vi "DB Manager.vi"(8 "error in":errorcluster caption="에러 입력(에러 없음)") -> (0 "error out":errorcluster caption="에러 출력")   [LabVIEW 2020]
uses:
  Support/Controls/Cmd_Mouse Popup.ctl
  Support/Controls/Clst_DBM data.ctl
  Support/Controls/Clst_Query Info.ctl
  <vilib>/Utility/miscctls.llb/LVRowAndColumnUnsignedTypeDef.ctl
  <vilib>/Utility/NIReport.llb/Report Type.ctl
  Support/Controls/Cmd_Read Query.ctl
  Support/Controls/Cmd_Write Query.ctl
  Variables/Global_Cal Info.vi
  Support/Public/Polymorph/Cell Space_ListBox.vi
  Support/Public/Polymorph/Data Class_2D Str.vi
  Support/Public/Polymorph/Cell Space_Table.vi
  <vilib>/Utility/error.llb/Error Cluster From Error Code.vi
  <vilib>/addons/_office/excel.llb/Excel Get Data (str).vi
  Support/Public/Polymorph/Array Dedup_1D Str.vi
  <vilib>/ErrorRing/Error Ring.xnode
  <vilib>/addons/database/NI_Database_API.lvlib
  <vilib>/Utility/NIReport.llb/NI_report.lvclass
  <vilib>/Utility/NIReport.llb/NI_ReportGenerationCore.lvlib
  <vilib>/addons/_office/NI_ReportGenerationToolkit.lvlib
  <vilib>/Utility/NIReport.llb/Excel/NI_Excel.lvclass
panel:
  out "Data":string[][](array[string])
  out "모델등록요청":u8
  out "기준기등록요청":u8
  in  "TOP_요청삭제":bool
  in  "TOP_등록요청":bool
  in  "TOP_추가":bool
  in  "TOP_항목명":u16(ring) caption="항목명" items=["ALL [ - ]", "10201-0 [ 볼; 강구, 표준구 등 ]", "10203-0 [ 기계/전기식 콤퍼레이터 ]", "10206-0 [ 다이얼/실린더 게이지 시험기 ]", "10207-0 [ 닥터 블레이드 ]", "10209-0 [ 엔드바, 마이크로미터 기준봉 ]", "10210-1 [ 길이 변위계 ]", "10210-2 [ LVDT ]", "10211-0 [ 틈새 게이지 ]", "10212-0 [ 필름 어플리케이터 ]", "10213-0 [ 갭 게이지 ]", "10214-0 [ 게이지 블록, 비교교정 ]", "10216-0 [ 높이 게이지/측정기 ]", "10219-0 [ 리니어 스케일 ]", "10220-0 [ 표준 측장기 ]", "10223-0 [ 전기 마이크로미터 ]", "10224-1 [ 높이 마이크로미터 ]", "10224-2 [ 받침블록 ]", "10225-0 [ 레이저 스캔 마이크로미터 ]", "10227-0 [ 표준 내/외경 줄자 ]", "10228-1 [ 원통형 플러그 게이지 ]", "10228-2 [ 핀 게이지 ]", "10229-0 [ 래디어스 게이지 ]", "10230-0 [ 원통형 링 게이지 ]", "10231-0 [ 게이지 블록 단차시편 ]", "10232-1 [ 스텝 게이지 ]", "10232-2 [ 캘리퍼 검사기 ]", "10233-0 [ 테이퍼형 틈새 게이지 ]", "10234-0 [ 초음파식 두께 측정기 ]", "10235-1 [ 두께 측정용 기준시편; 코팅형 ]", "10235-2 [ 두께 측정용 기준시편; 초음파 시편 ]", "10236-0 [ 피막 두께 측정기 ]", "10237-0 [ 토크 암 ]", "10238-0 [ 폭 측정용 기준 시편 ]", "10304-1 [ 각도정규 ]", "10304-2 [ 디지털 각도기 ]", "10311-1 [ 전기식 수준기 ]", "10311-2 [ 평형/각형 수준기 ]", "10317-0 [ 사인바, 플레이트, 테이블, 센터 ]", "10318-0 [ 직각도 시험기 ]", "10319-0 [ 원통 스퀘어 ]", "10320-0 [ 정밀직각기준, 직각자 ]", "10401-0 [ 형상 측정기 ]", "10404-0 [ 옵티컬 플랫 ]", "10405-0 [ 옵티컬 파라렐 ]", "10406-0 [ 평행블록 ]", "10407-0 [ 정밀 정반 ]", "10409-0 [ 진원도 측정기 ]", "10412-0 [ 스트레이트 엣지 ]", "10413-0 [ 곧은자 ]", "10415-0 [ 테스트 바아 ]", "10416-0 [ 구면계 ]", "10503-0 [ 접촉식 좌표 측정기 ]", "10504-1 [ 비접촉식 좌표 측정기 ]", "10504-2 [ 화상측정기 ]", "10505-0 [ 게이지 블록 부속품 ]", "10511-1 [ 측정현미경 ]", "10511-2 [ 측정투영기 ]", "10511-3 [ 측정 현미경 (영상) ]", "10512-0 [ 측미 현미경 ]", "10517-0 [ 촉침식 표면 거칠기 측정기 ]", "10525-0 [ 나사 플러그 게이지 ]", "10529-0 [ 브이블록 및 박스블록 ]", "10601-1 [ 내/외측 캘리퍼 ]", "10601-3 [ 캘리퍼 게이지 ]", "10603-1 [ 실린더 게이지 ]", "10603-2 [ 보어 게이지 ]", "10604-1 [ 깊이 게이지 ]", "10604-2 [ 깊이마이크로미터 ]", "10605-1 [ 다이얼/디지털 게이지 ]", "10605-2 [ 다이얼 및 디지털 두께 측정기 ]", "10609-1 [ 지침 측미기 ]", "10609-2 [ 테스트 인디케이터 ]", "10610-0 [ 마이크로미터 헤드 ]", "10611-0 [ 3점 마이크로미터 ]", "10612-1 [ 내측 마이크로미터 ]", "10612-2 [ 봉형 내측 마이크로미터 ]", "10613-1 [ 외측 마이크로미터 ]", "10613-2 [ V-앤빌 마이크로미터 ]", "10613-3 [ 벤치 마이크로미터 ]", "10615-1 [ 공기입자계수기 ]", "10615-2 [ 액체 입자계수기 ]", "10617-0 [ 표준체 ]", "10620-0 [ 용접 게이지 ]", "10622-0 [ 입자희석장치 ]", "20105-0 [ 부등비 접시 수동 저울 ]", "20106-0 [ 판 지시 저울 ]", "20108-0 [ 반 지시 맞 저울 ]", "20109-0 [ 전기식 지시 저울 ]", "20112-0 [ 판수동/플랫트 폼 저울 ]", "20113-0 [ 접시 지시저울,스프링 지시 저울 ]", "20116-1 [ 분동 ]", "20116-2 [ 추 ]", "20202-0 [ 힘 측정기 ]", "20203-0 [ 인장 및 압축 시험기 ]", "20204-0 [ 푸쉬풀 게이지 ]", "20302-0 [ 토크 측정기 ]", "20303-0 [ 토크 렌치 및 토크 드라이버 ]", "20402-0 [ 액주형 압력계 ]", "20406-0 [ 절대압계 ]", "20408-0 [ 연성 압력계 ]", "20409-0 [ 차압계 ]", "20411-1 [ 게이지압용 압력계 ]", "20411-2 [ AUTOCLAVE, HAST CHAMBER(지시계포함) ]", "20411-3 [ 압력조절기 ]", "20411-4 [ 압력기록계 ]", "20412-1 [ 압력 변환기/전송기(게이지압) ]", "20412-2 [ 압력 변환기/전송기(절대압) ]", "20412-3 [ 압력 변환기/전송기(차압) ]", "20413-0 [ 다이얼형 진공계 ]", "20414-0 [ 수심계 ]", "20601-0 [ 유리제 부피계; 타 재질 포함 ]", "20602-0 [ 비중병; 스테인리스 스틸 포함 ]", "20605-0 [ 콘크리트 공기량 시험기 ]", "20606-0 [ 피스톤식 부피계 ]", "20802-0 [ 회전형 점도계 ]", "20901-1 [ 열선형 유속계 ]", "20901-2 [ 열선형 유속계(센서형) ]", "20902-0 [ 피토관 유속계 ]", "20908-0 [ 기체용 차압 유량계 ]", "20909-0 [ 액체용 차압 유량계 ]", "20910-0 [ 액체용 전자기 유량계 ]", "20911-0 [ 기체용 질량 유량계 ]", "20912-0 [ 액체용 질량 유량계 ]", "20914-0 [ 기체용 용적 유량계 ]", "20915-0 [ 액체용 용적 유량계 ]", "20916-0 [ 기체용 터빈 유량계 ]", "20917-0 [ 액체용 터빈 유량계 ]", "20918-0 [ 기체용 초음파 유량계 ]", "20919-0 [ 액체용 초음파 유량계 ]", "20920-0 [ 기체용 면적 유량계 ]", "20921-0 [ 액체용 면적 유량계 ]", "20922-0 [ 기체용 와 유량계 ]", "20923-0 [ 액체용 와 유량계 ]", "20925-0 [ 회전형 유속계 ]", "30102-1 [ 주파수 표준기 ]", "30102-2 [ 주파수 비교기 ]", "30103-0 [ 주파수 발생기 ]", "30104-1 [ 주파수 계수기 ]", "30104-2 [ 주파수 계수기 플러그 유니트 ]", "30104-3 [ 상용 주파수계 ]", "30104-4 [ 주파수 계 ]", "30105-1 [ 시간간격 발생기 ]", "30105-2 [ 주파수 발생기 ]", "30106-1 [ 시간간격 측정기 ]", "30106-2 [ 초시계 ]", "30106-3 [ 타이머 ]", "30106-4 [ 카운터 ]", "30201-0 [ 표준 회전속도 발생장치 ]", "30202-0 [ 접촉식 회전 속도계 ]", "30203-0 [ 광 회전 속도계 ]", "30205-0 [ 와우-후러터 발생장치 ]", "30206-0 [ 와우-후러터 미터 ]", "40101-0 [ 직류 전류계 ]", "40102-0 [ 직류 전압전류 변환기 ]", "40103-0 [ 직류 전압/전류 교정기 ]", "40104-0 [ 전기식 온도 교정기 ]", "40105-0 [ 직류용 분류기 ]", "40106-0 [ 검류계 ]", "40108-0 [ 직류 전원 공급기 ]", "40110-0 [ 직류 전압 분할기 ]", "40111-0 [ 전자형 직류 기준전압 ]", "40112-1 [ 직류 전압계 ]", "40112-2 [ 차동 전압계 등 ]", "40113-1 [ 정전기 측정기 ]", "40113-2 [ 이온 측정기 ]", "40201-1 [ 용량 브리지 ]", "40201-2 [ 용량 지시기 ]", "40202-0 [ 계단식 용량기 ]", "40204-0 [ 표준 용량기 ]", "40205-0 [ 접지 저항 측정기 ]", "40208-1 [ 유도기 ]", "40208-2 [ 계단식 유도기 ]", "40210-0 [ 절연시험기 ]", "40211-0 [ Q-미터 ]", "40213-1 [ 저항 브리지 ]", "40213-2 [ 저항 유사장비 ]", "40214-0 [ 저항 측정기 ]", "40215-1 [ 표준 저항기 ]", "40215-2 [ 계단식 저항기 ]", "40216-1 [ 전기전도도 미터 ]", "40216-2 [ 전도도 미터 ]", "40217-1 [ LCR 미터 ]", "40217-2 [ 임피던스 브리지 ]", "40301-0 [ 교류 전류계 ]", "40302-1 [ 클램프형  전류계/전압계 ]", "40302-2 [ 전류코일 ]", "40303-0 [ 교류 전압/전류 교정기 ]", "40304-0 [ 전력계 교정기 ]", "40305-0 [ 교류 전류 분류기 ]", "40310-1 [ 역률계 ]", "40310-2 [ 무효율계 ]", "40311-0 [ 교류 전력계 ]", "40312-0 [ 교류 전원 공급기 ]", "40313-0 [ 내전압/전기 안전 시험기 ]", "40314-0 [ 전력 기록계 ]", "40318-0 [ 교류 전압계/전위차, 실효치 ]", "40401-1 [ 저주파 증폭기 ]", "40401-2 [ 챠지/전압 증폭기 ]", "40402-0 [ 직류/저주파 감쇠기 ]", "40403-0 [ 멀티미터 교정기 ]", "40404-0 [ 파형 측정기 교정기 ]", "40406-0 [ 영상 신호 발생기 ]", "40407-1 [ 오디오 분석기 ]", "40407-2 [ 왜율 미터 ]", "40408-0 [ 저주파용 여파기 ]", "40409-0 [ 저주파 신호 분석기 ]", "40410-0 [ 전원 주파수계 ]", "40411-1 [ 다기능 파형 발생기 ]", "40411-2 [ 구형파 발생기 ]", "40412-0 [ 제네스코프 ]", "40413-0 [ 직·교류 고전압계 ]", "40416-0 [ 누설전류 시험기 ]", "40417-0 [ 직/교류 전자부하 ]", "40419-0 [ 멀티미터 ]", "40420-0 [ 잡음 전압 측정기 ]", "40421-0 [ 파형 측정기 ]", "40422-0 [ 저주파 위상계 ]", "40423-0 [ 랜덤파형 발생기 ]", "40424-0 [ 전압 전류 기록계 ]", "40425-0 [ 릴레이 시험기 ]", "40426-0 [ LF 신호 발생기 ]", "40427-0 [ 저주파 스펙트럼 분석기 ]", "40429-0 [ 스위프 발생기 ]", "40432-0 [ 트란지스터 특성 곡선 측정기 ]", "40433-0 [ 파형 분석기 ]", "40434-0 [ 직/교류 고전압 출력기 ]", "40435-0 [ 직/교류 고전압 프로브 ]", "40436-0 [ 논리 회로분석기 ]", "40437-0 [ 전화기 시험기 ]", "40438-0 [ 영상 신호 분석기 ]", "40503-0 [ 자속 미터 ]", "40504-0 [ 플럭스 원 ]", "40508-0 [ 마그네토 미터 ]", "40510-0 [ 표준 자석 ]", "40601-0 [ 고주파 증폭기 ]", "40602-1 [ 동축형 고정 감쇠기 ]", "40602-2 [ 동축형 가변 감쇠기 ]", "40603-1 [ 도파관형 고정 감쇠기 ]", "40603-2 [ 도파관형 가변 감쇠기 ]", "40605-0 [ 버스트 펄스 발생기 ]", "40606-0 [ 감쇠기 교정기 ]", "40607-0 [ 고주파 전력 측정기 교정기 ]", "40608-1 [ EMC용 변환기 ]", "40608-2 [ 흡수 클램프 ]", "40610-0 [ 동축형 방향성 결합기/분배기 ]", "40611-0 [ 도파관형 방향성 결합기 ]", "40613-0 [ 정전기 발생기 ]", "40614-0 [ EMC 수신기 ]", "40615-0 [ 고주파/전자파 여파기 ]", "40616-0 [ 고주파 임피던스 미터 ]", "40617-0 [ 고주파 스펙트럼 분석기 ]", "40618-1 [ 전원 임피던스 안정화 회로망 ]", "40618-2 [ 결합 감결합 회로망 ]", "40618-3 [ 임피던스 안정화 회로망 ]", "40618-4 [ 전자기 클램프 ]", "40618-5 [ 임피던스 변환기 ]", "40619-1 [ 동축형 표준 부정합 ]", "40621-0 [ 이동통신 종합시험기 ]", "40622-0 [ 변조계 ]", "40623-0 [ 회로망 분석기 ]", "40624-0 [ 잡음계수 측정기 ]", "40625-0 [ 잡음 발생기 ]", "40626-0 [ 잡음 충격파 시험기 ]", "40635-1 [ 고주파 전력 측정기 ]", "40635-2 [ 고주파 고전력계 ]", "40636-0 [ 다이오드 전력 감지기 ]", "40637-0 [ 열전대 전력 감지기 ]", "40638-0 [ 펄스 발생기 ]", "40639-1 [ 레이더 시험장치 ]", "40639-2 [ 레이더 시험장치 ]", "40639-3 [ 레이더 시험장치 ]", "40639-4 [ 레이더 시험장치 ]", "40639-5 [ 레이더 시험장치 ]", "40640-0 [ 고주파 신호 발생기 ]", "40641-1 [ 고주파 스펙트럼 분석기 ]", "40641-2 [ FFT 분석기 ]", "40642-0 [ 속도 측정기 ]", "40643-0 [ 서지 발생기 ]", "40645-0 [ 고주파 터미네이션 ]", "40646-0 [ 동축형 서미스터 마운트 ]", "40648-0 [ 전송 장애 측정 시험기 ]", "40650-0 [ 고주파 전압계 ]", "40651-0 [ 벡터 전압계 ]", "40652-0 [ 전자기장의 세기 측정기 ]", "40653-0 [ 측정 수신기 ]", "40654-0 [ 딥 시뮬레이터 ]", "40701-0 [ 누설 전자파 측정기 ]", "40702-1 [ 프로브 류-전계 프로브 ]", "40702-2 [ 프로브 류-자계 프로브 ]", "40703-1 [ 이극 안테나 류-SAR 측정용 전기장 프로브 ]", "40703-2 [ 이극 안테나 류-SAR 측정용 다이폴 안테나 ]", "40703-3 [ 이극 안테나 류-다이폴 안테나 ]", "40703-4 [ 이극 안테나 류-바이코니컬 안테나 ]", "40703-5 [ 이극 안테나 류-대수주기 안테나 ]", "40703-6 [ 이극 안테나 류-하이브리드 안테나 ]", "40704-0 [ 환상 안테나 류 ]", "40705-0 [ 단극 안테나 류 ]", "40707-0 [ 혼 안테나 류 ]", "50101-1 [ 온도 조절형 챔버 및 오븐 ]", "50101-2 [ 전기로 ]", "50101-3 [ 액체항온조 ]", "50101-4 [ 빙점조 ]", "50101-5 [ 드라이블럭교정기 ]", "50102-1 [ 온도 지시계(센서포함_열전식) ]", "50102-2 [ 온도 지시계(센서미포함_열전식) ]", "50102-3 [ 온도 지시계(센서미포함_저항식) ]", "50102-4 [ 온도 지시계(센서포함_저항식) ]", "50103-0 [ 유리제 온도계 ]", "50104-0 [ 저항식 온도계 ]", "50105-0 [ 열팽창식 온도계 ]", "50106-1 [ 열전대(귀금속) ]", "50106-2 [ 열전대(비금속) ]", "50107-0 [ 온도 변환기 ]", "50204-0 [ 복사온도계 ]", "50205-0 [ 복사열 영상측정장치 ]", "50206-0 [ 흑체로 ]", "50301-0 [ 알루미나 박막습도계 ]", "50302-1 [ 고분자 박막습도계 ]", "50302-2 [ 모발 습도계 ]", "50302-3 [ 디지털온습도계 ]", "50304-0 [ 온도/습도 기록계 ]", "50305-0 [ 상대습도 변환기 ]", "50306-1 [ 분류식 습도발생장치 ]", "50306-2 [ 항온항습기 ]", "60102-1 [ 다기능 음향 교정기 ]", "60102-2 [ 피스톤폰 ]", "60102-3 [ 음압 레벨교정기 ]", "60104-1 [ 마이크로폰 ]", "60104-2 [ 마이크로폰(3단자 결합기) ]", "60106-1 [ 소음계 ]", "60106-2 [ 소음계 ]", "60301-0 [ 진동계 교정기 ]", "60302-1 [ 진동 변환기 ]", "60302-2 [ 충격 변환기 ]", "60303-1 [ 진동 측정기 ]", "60303-2 [ 충격 측정기 ]", "70101-0 [ 광조도계 ]", "70102-0 [ 광휘도계 ]", "70103-0 [ 전광선속계 ]", "70104-0 [ 광도계 ]", "70202-0 [ 색온도측정기 ]", "70203-0 [ 색온도 표준전구 ]", "70204-0 [ 색채계; 광원색 ]", "70209-0 [ 전광선속 표준전구 ]", "70213-0 [ 디스플레이 색채 분석기; 광휘도, 색좌표, 화이트밸런스 등 ]", "70214-0 [ 광도 표준전구 ]", "70215-0 [ 분광복사조도 표준전구 ]", "70216-0 [ 전분광복사선속 표준전구 ]", "70217-0 [ 광휘도 표준광원 ]", "70218-0 [ 분광복사휘도 표준광원 ]", "70219-0 [ 자외선 복사조도계 ]", "70220-0 [ 분광복사조도계 ]", "70221-0 [ 전분광복사선속계 ]", "70222-0 [ 분광복사휘도계 ]", "70223-0 [ 분광복사도계 ]", "70402-0 [ 광대역광원 ]", "70410-0 [ 광감쇠기 ]", "70413-0 [ 광감쇠량측정기 ]", "70415-0 [ 광 멀티미터 ]", "70417-0 [ 광스펙트럼 분석기 ]", "70418-0 [ 시간영역 광반사계 ]", "70430-0 [ ASE 광원 ]", "70433-0 [ 광출력 안정화 레이저 및 LDs ]", "90102-0 [ 대기가스 감시기 ]", "90103-0 [ 가스 분석기 ]", "90104-0 [ 배기가스 측정기 ]", "N0001-0 [ INSPECTION JIG & FIXTURE ]", "N0002-0 [ 진동시험기 ]"]
  in  "TOP_삭제":bool
  in  "TOP_파일생성":bool
  in  "TOP_등록":bool
  in  "TOP_조회":bool
  in  "TOP_초기화":bool
  in  "TOP_종료":bool
  out "Func":string
  out "SubVI List":string[](array[string])
  out "슬라이드":u32(slide) scale=-1.0..3.0
  out "교정기능목록":string[][](array[string])
  out "세부분류목록":string[][](array[string])=[["ALL", "-"], ["10201-0", "볼; 강구, 표준구 등"], ["10206-0", "다이얼/실린더 게이지 시험기"], ["10209-0", "엔드바, 마이크로미터 기준봉"], ["10210-1", "길이 변위계"], ["10210-2", "LVDT"], ["10210-3", "길이 변위계"], ["10211-0", "틈새 게이지"], ["10213-0", "갭 게이지"], ["10214-0", "게이지 블록, 비교교정"], ["10216-0", "높이 게이지/측정기"], ["10220-0", "표준 측장기"], ["10223-0", "전기 마이크로미터"], ["10224-1", "높이 마이크로미터"], ["10224-2", "받침블록"], ["10227-0", "표준 내/외경 줄자"], ["10228-1", "원통형 플러그 게이지"], ["10228-2", "핀 게이지"], ["10229-0", "래디어스 게이지"], ["10230-0", "원통형 링 게이지"], ["10232-1", "스텝 게이지"], ["10232-2", "캘리퍼 검사기"], ["10233-0", "테이퍼형 틈새 게이지"], ["10234-0", "초음파식 두께 측정기"], ["10235-0", "두께 측정용 기준시편;코팅형, 초음파 시편"], ["10236-0", "피막 두께 측정기"], ["10304-1", "각도정규"], ["10304-2", "콤비네이션셋"], ["10311-1", "전기식 수준기"], ["10311-2", "평형/각형 수준기"], ["10404-0", "옵티컬 플랫"], ["10405-0", "옵티컬 파라렐"], ["10407-0", "정밀 정반"], ["10413-0", "곧은자"], ["10503-0", "접촉식 좌표 측정기"], ["10504-0", "비접촉식 좌표 측정기"], ["10511-1", "측정현미경"], ["10511-2", "측정투영기"], ["10511-3", "측정 현미경 (영상)"], ["10512-0", "측미 현미경"], ["10525-0", "나사 플러그 게이지"], ["10601-1", "내/외측 캘리퍼"], ["10601-3", "캘리퍼 게이지"], ["10603-1", "실린더 게이지"], ["10603-2", "보어 게이지"], ["10604-1", "깊이 게이지"], ["10604-2", "깊이마이크로미터"], ["10605-0", "다이얼/디지털 게이지"], ["10609-1", "지침 측미기"], ["10609-2", "테스트 인디케이터"], ["10610-0", "마이크로미터 헤드"], ["10611-0", "3점 마이크로미터"], ["10612-1", "내측 마이크로미터"], ["10612-2", "봉형 내측 마이크로미터"], ["10613-1", "외측 마이크로미터"], ["10615-1", "공기입자계수기"], ["10615-2", "액체 입자계수기"], ["10617-0", "표준체"], ["10620-0", "용접 게이지"], ["10622-0", "입자희석장치"], ["20105-0", "부등비 접시 수동 저울"], ["20108-0", "반 지시 맞 저울"], ["20109-0", "전기식 지시 저울"], ["20112-0", "판수동/플랫트 폼 저울"], ["20113-0", "접시 지시저울,스프링 지시 저울"], ["20116-1", "분동"], ["20116-2", "추"], ["20202-0", "힘 측정기"], ["20203-0", "인장 및 압축 시험기"], ["20204-0", "푸쉬풀 게이지"], ["20302-0", "토크 측정기"], ["20303-0", "토크 렌치 및 토크 드라이버"], ["20406-0", "절대압계"], ["20408-0", "연성 압력계"], ["20409-0", "차압계"], ["20411-1", "게이지압용 압력계"], ["20411-2", "압력 발생기"], ["20411-3", "압력 조절기"], ["20411-4", "압력기록계"], ["20412-0", "압력 변환기/전송기"], ["20413-0", "다이얼형 진공계"], ["20414-0", "수심계"], ["20901-1", "열선형 유속계"], ["20901-2", "열선형 유속계(센서형)"], ["20902-0", "피토관 유속계"], ["20925-0", "회전형 유속계"], ["30102-1", "주파수 표준기"], ["30102-2", "주파수 비교기"], ["30103-0", "주파수 발생기"], ["30104-1", "주파수 계수기"], ["30104-2", "주파수 계수기 플러그 유니트"], ["30104-3", "상용 주파수계"], ["30104-4", "주파수 계"], ["30105-1", "시간간격 발생기"], ["30105-2", "주파수 발생기"], ["30106-1", "시간간격 측정기"], ["30106-2", "초시계"], ["30106-3", "타이머"], ["30201-0", "표준 회전속도 발생장치"], ["30202-0", "접촉식 회전 속도계"], ["30203-0", "광 회전 속도계"], ["30205-0", "와우-후러터 발생장치"], ["30206-0", "와우-후러터 미터"], ["40101-0", "직류 전류계"], ["40102-0", "직류 전압전류 변환기"], ["40103-0", "직류 전압/전류 교정기"], ["40104-0", "전기식 온도 교정기"], ["40105-0", "직류용 분류기"], ["40106-0", "검류계"], ["40108-0", "직류 전원 공급기"], ["40111-0", "전자형 직류 기준전압"], ["40112-1", "직류 전압계"], ["40112-2", "차동 전압계 등"], ["40113-1", "정전기 측정기"], ["40113-2", "이온 측정기"], ["40201-1", "용량 브리지"], ["40201-2", "용량 지시기"], ["40202-0", "계단식 용량기"], ["40204-0", "표준 용량기"], ["40205-0", "접지 저항 측정기"], ["40208-1", "유도기"], ["40208-2", "계단식 유도기"], ["40210-0", "절연시험기"], ["40211-0", "Q-미터"], ["40213-1", "저항 브리지"], ["40213-2", "저항 유사장비"], ["40214-0", "저항 측정기"], ["40215-1", "표준 저항기"], ["40215-2", "계단식 저항기"], ["40216-1", "전기전도도 미터"], ["40216-2", "전도도 미터"], ["40217-1", "LCR 미터"], ["40217-2", "임피던스 브리지"], ["40301-0", "교류 전류계"], ["40302-1", "클램프형  전류계/전압계"], ["40302-2", "전류코일"], ["40303-0", "교류 전압/전류 교정기"], ["40305-0", "교류 전류 분류기"], ["40310-1", "역률계"], ["40310-2", "무효율계"], ["40311-0", "교류 전력계"], ["40312-0", "교류 전원 공급기"], ["40313-0", "내전압/전기 안전 시험기"], ["40314-0", "전력 기록계"], ["40318-0", "교류 전압계/전위차, 실효치"], ["40401-1", "저주파 증폭기"], ["40401-2", "챠지/전압 증폭기"], ["40402-0", "직류/저주파 감쇠기"], ["40403-0", "멀티미터 교정기"], ["40404-0", "파형 측정기 교정기"], ["40406-0", "영상 신호 발생기"], ["40407-1", "오디오 분석기"], ["40407-2", "왜율 미터"], ["40408-0", "저주파용 여파기"], ["40409-0", "저주파 신호 분석기"], ["40410-0", "전원 주파수계"], ["40411-1", "다기능 파형 발생기"], ["40411-2", "구형파 발생기"], ["40412-0", "제네스코프"], ["40413-0", "직·교류 고전압계"], ["40416-0", "누설전류 시험기"], ["40417-0", "직/교류 전자부하"], ["40419-0", "멀티미터"], ["40420-0", "잡음 전압 측정기"], ["40421-0", "파형 측정기"], ["40422-0", "저주파 위상계"], ["40423-0", "랜덤파형 발생기"], ["40424-0", "전압 전류 기록계"], ["40425-0", "릴레이 시험기"], ["40426-0", "LF 신호 발생기"], ["40427-0", "저주파 스펙트럼 분석기"], ["40429-0", "스위프 발생기"], ["40432-0", "트란지스터 특성 곡선 측정기"], ["40433-0", "파형 분석기"], ["40434-0", "직/교류 고전압 출력기"], ["40435-0", "직/교류 고전압 프로브"], ["40436-0", "논리 회로분석기"], ["40437-0", "전화기 시험기"], ["40438-0", "영상 신호 분석기"], ["40503-0", "자속 미터"], ["40504-0", "플럭스 원"], ["40508-0", "마그네토 미터"], ["40510-0", "표준 자석"], ["40601-0", "고주파 증폭기"], ["40602-1", "동축형 고정 감쇠기"], ["40602-2", "동축형 가변 감쇠기"], ["40605-0", "버스트 펄스 발생기"], ["40606-0", "감쇠기 교정기"], ["40607-0", "고주파 전력 측정기 교정기"], ["40608-1", "EMC용 변환기"], ["40608-2", "흡수 클램프"], ["40610-0", "동축형 방향성 결합기/분배기"], ["40613-0", "정전기 발생기"], ["40614-0", "EMC 수신기"], ["40615-0", "고주파/전자파 여파기"], ["40616-0", "고주파 임피던스 미터"], ["40617-0", "고주파 스펙트럼 분석기"], ["40618-1", "전원 임피던스 안정화 회로망"], ["40618-2", "결합 감결합 회로망"], ["40618-3", "임피던스 안정화 회로망"], ["40618-4", "전자기 클램프"], ["40618-5", "임피던스 변환기"], ["40619-1", "동축형 표준 부정합"], ["40621-0", "이동통신 종합시험기"], ["40622-0", "변조계"], ["40623-0", "회로망 분석기"], ["40624-0", "잡음계수 측정기"], ["40625-0", "잡음 발생기"], ["40626-0", "잡음 충격파 시험기"], ["40635-1", "고주파 전력 측정기"], ["40635-2", "고주파 고전력계"], ["40636-0", "다이오드 전력 감지기"], ["40637-0", "열전대 전력 감지기"], ["40638-0", "펄스 발생기"], ["40639-0", "레이더 시험장치"], ["40640-0", "고주파 신호 발생기"], ["40641-1", "고주파 스펙트럼 분석기"], ["40641-2", "FFT 분석기"], ["40642-0", "속도 측정기"], ["40643-0", "서지 발생기"], ["40645-0", "고주파 터미네이션"], ["40646-0", "동축형 서미스터 마운트"], ["40648-0", "전송 장애 측정 시험기"], ["40650-0", "고주파 전압계"], ["40651-0", "벡터 전압계"], ["40652-0", "전자기장의 세기 측정기"], ["40653-0", "측정 수신기"], ["40654-0", "딥 시뮬레이터"], ["40702-1", "프로브 류-전계 프로브"], ["40702-2", "프로브 류-자계 프로브"], ["40703-1", "이극 안테나 류-SAR 측정용 전기장 프로브"], ["40703-2", "이극 안테나 류-SAR 측정용 다이폴 안테나"], ["40703-3", "이극 안테나 류-다이폴 안테나"], ["40703-4", "이극 안테나 류-바이코니컬 안테나"], ["40703-5", "이극 안테나 류-대수주기 안테나"], ["40703-6", "이극 안테나 류-하이브리드 안테나"], ["40704-0", "환상 안테나 류"], ["40705-0", "단극 안테나 류"], ["40707-0", "혼 안테나 류"], ["50101-1", "온도 조절형 챔버 및 오븐"], ["50101-2", "전기로"], ["50101-3", "액체항온조"], ["50101-4", "빙점조"], ["50101-5", "드라이블럭교정기"], ["50102-1", "온도 지시계(센서포함)"], ["50102-2", "온도 지시계(센서미포함_열전식)"], ["50102-3", "온도 지시계(센서미포함_저항식)"], ["50103-0", "유리제 온도계"], ["50104-0", "저항식 온도계"], ["50105-0", "열팽창식 온도계"], ["50106-1", "열전대(귀금속)"], ["50106-2", "열전대(비금속)"], ["50107-0", "온도 변환기"], ["50204-0", "복사온도계"], ["50301-0", "알루미나 박막습도계"], ["50302-1", "고분자 박막습도계"], ["50302-2", "모발 습도계"], ["50302-3", "디지털온습도계"], ["50304-0", "온도/습도 기록계"], ["50305-0", "상대습도 변환기"], ["50306-1", "분류식 습도발생장치"], ["50306-2", "항온항습기"], ["60102-1", "다기능 음향 교정기"], ["60102-2", "피스톤폰"], ["60102-3", "음압 레벨교정기"], ["60104-0", "마이크로폰"], ["60106-1", "소음계"], ["60106-2", "소음계"], ["60301-0", "진동계 교정기"], ["60302-0", "진동 변환기"], ["60303-0", "진동 측정기"], ["70101-0", "광조도계"], ["70418-0", "시간영역 광반사계"], ["90103-0", "가스 분석기"]]
  in  "탭 컨트롤":T1(tab)
  in  "STD_temp_LIST":i32(listbox)
  in  "STD_DB요청리스트":bool
  in  "STD_다시열기":bool
  out "STD Update":string caption="업데이트 일시"
  in  "파일닫기?":bool=TRUE
  in  "STD_notuse":bool caption="사용여부"
  in  "STD_DB 내용 검토":bool
  in  "STD_List box":i32(listbox)
  in  "STD_등록List 검색":bool
  out "Cal Date ok?":bool caption="교정일자일치?"
  in  "STD_교정일자":string(combo) caption="교정일자"
  out "STDDB ok?":bool caption="등록 가능?"
  in  "STD_File Path":path caption="기준기 성적서 Excel 파일 경로"
  in  "ISID":string caption="등록번호"
  in  "TBCALSTD":string[][](table)
  in  "STDDB STD List":string(combo) caption="기준기명"
  in  "STD_DB오류목록":bool
  in  "PROC_지우기 2":bool
  in  "PROC_지우기 1":bool
  in  "PROC_절차생성":bool
  in  "PROC_새로고침":bool
  in  "옵션":string
  in  "PROC_모델 선택":string(combo) caption="모델 선택"
  in  "PROC MDL":string caption="모델명"
  in  "PROC_모델 검색":bool
  in  "PROC_등록요청LIST":i32(listbox)
  in  "TBCALPROC":string[][](table)
  in  "TBCALFUNC":string[][](table)
  out "Func Ind":string caption="교정기능"
  out "Func List tbl":string[][](array[string])
  in  "STD List":string(combo) caption="기준기명"
  in  "USE_STD 추가":bool
  in  "USE_Func_ext":string(combo) caption="세부교정기능"
  in  "TBUSESTD":string[][](table)
  in  "TBCALNAME":string[][](table)
  in  "STDNAM List":string(combo) caption="기준기명"
  in  "TBSTDNAME":string[][](table)
  in  "TBCALCMC":string[][](table)
  out "CMC Update":string caption="업데이트 일시"
  in  "TBCALSPEC":string[][](table)
  # "0 : 사용, 1 : 미사용"
  # "※ 기준기 DB 등록시, 2번 등록됨."
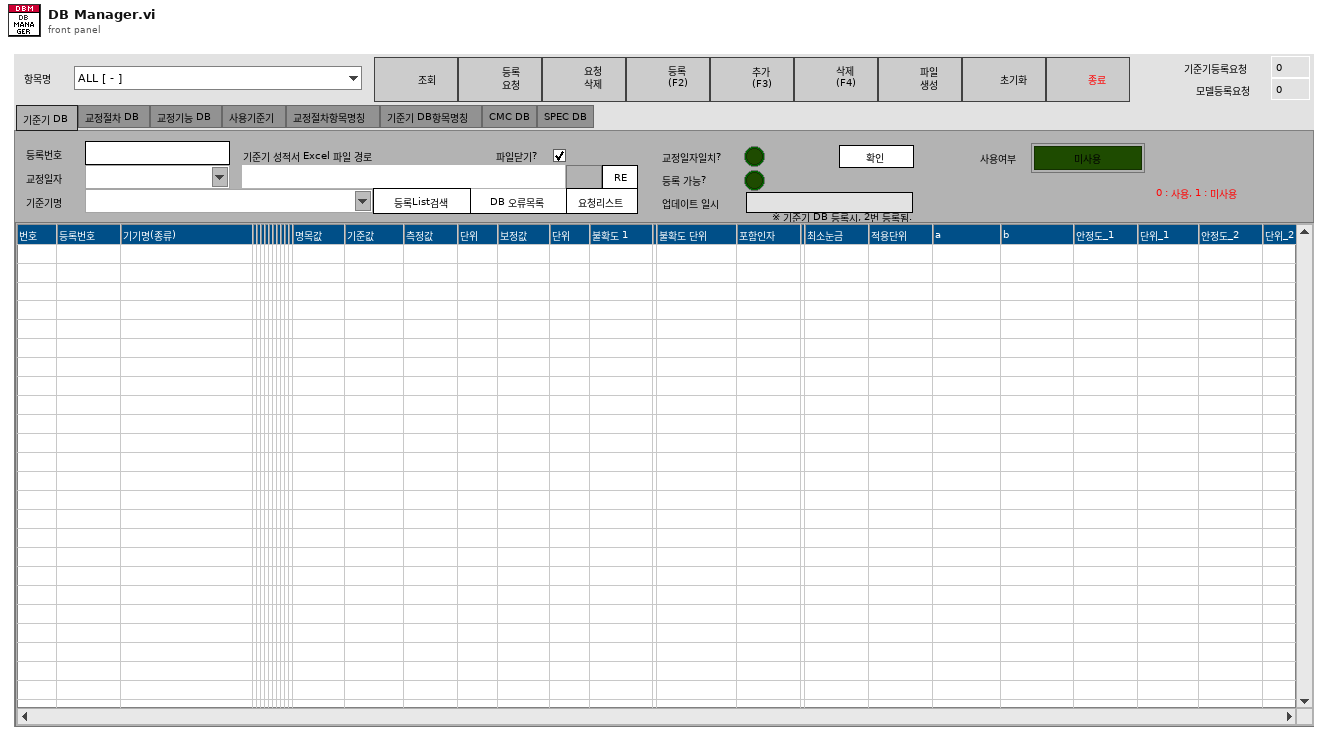
[diagram p1: front panel]
types:
  T1 = enum32{"기준기 DB", "교정절차 DB", "교정기능 DB", "사용기준기", "교정절차항목명칭", "기준기 DB항목명칭", "CMC DB", "SPEC DB"}
  T2 = cluster{"세부분류코드":string, "형식":string, "옵션":string, "측정기명":string, "EXCEL파일명":string, "TEMP":string}
  T3 = typedef "Cmd_Mouse Popup.ctl" = enum16{"활성화", "메뉴선택"}
  T4 = typedef "Clst_DBM data.ctl" = cluster{"문자열":string, "불리언":bool, "원소":refnum<vi>}
  T5 = cluster{"Shift":bool, "Ctrl":bool, "Alt":bool, "Cmd":bool, "Opt":bool}
  T6 = enum8{"Enabled", "Disabled", "Disabled and Grayed Out"}
  T7 = typedef "Clst_Query Info.ctl" = cluster{"사번":string, "등록번호":string, "업체명":string, "세부분류코드":string, "형식":string, "기기번호":string, "FUNC":string, "FUNC_EXT":string, "옵션":string, "추가문자열":string, "일자":string, "배열 1":string[], "배열 2":string[], "항목명":string, "문자열":string, "이름":string}
  T8 = typedef "LVRowAndColumnUnsignedTypeDef.ctl" = cluster{"Row":u32, "Column":u32}
  T9 = typedef "NI_ReportGenerationCore.lvlib/Report Type.ctl" = enum16{"HTML", "Word", "Excel"}
  T10 = enum16{"maximized", "minimized", "normal", "no change"}
  T11 = typedef "Cmd_Read Query.ctl" = enum16{"교정자 이름 얻기", "인증교정자 얻기", "기술책임자 얻기", "기책부책 얻기", "등록번호 얻기", "등록정보 얻기", "업체정보 얻기", "교정일자(CAMAS) 얻기", "교정일자(CALSTD) 얻기", "교정환경 얻기", "교정절차서 목록 얻기", "교정절차서명 얻기", "교정절차 목록얻기", "교정절차 얻기", "PROC 교정절차 얻기", "PROC SPEC 얻기", "교정절차(Func별) 얻기", "교정절차(Func_ext별) 얻기", "기관코드 얻기", "교정기능(세부분류) 얻기", "교정기능(모델) 얻기", "교정기능 목록 얻기", "교정기능 명칭 얻기", "교정기능 항목명칭 얻기", "DB (사용기준기) 얻기", "DB (기준기이름) 얻기", "DB (기준기이름목록) 얻기", "DB (기준기목록) 얻기", "DB (기준기값) 얻기", "DB (CMC) 얻기", "DB (FUNC) 얻기", "DB (CALNAME) 얻기", "DB (STDNAME) 얻기", "DB (SPEC) 얻기", "모델(항목전체) 얻기", "모델(최대범위) 얻기", "모델(최소범위) 얻기", "모델(최대최소) 얻기", "모델(범위조건) 얻기", "모델(등록요청) 얻기", "모델(형식별) 얻기", "모델(조건별) 얻기", "모델(모델검색) 얻기", "세부분류 목록 얻기", "기준기등록리스트 얻기", "STD Cal Date Check", "DB등록일자 얻기", "적용항목 얻기", "기타정보 얻기", "기준기요청 얻기", "서버버전 얻기"}
  T12 = typedef "Cmd_Write Query.ctl" = enum16{"TBUSESTD_MCT Insert", "TBUSESTD_MCT Delete", "TBCALSTD_MCT_TEMP Insert", "TBCALSTD_MCT_TEMP Delete", "TBCALSTD_MCT Insert", "TBCALSTD_MCT Delete", "TBCALSTD_MCT_BACK Insert", "TBCALSTD_MCT_BACK Delete", "TBCALPROC_MCT Insert", "TBCALPROC_MCT Delete", "TBCALPROC_MCT_TEMP Insert", "TBCALPROC_MCT_TEMP Delete", "TBCALCMC_MCT Insert", "TBCALCMC_MCT Delete", "TBCALFUNC_MCT Insert", "TBCALFUNC_MCT Delete", "TBCALNAME_MCT Insert", "TBCALNAME_MCT Delete", "TBSTDNAME_MCT Insert", "TBSTDNAME_MCT Delete", "TBCALSPEC_MCT Insert", "TBCALSPEC_MCT Delete", "TBCALSTD_MCT NOTUSE update", "TBCALSPEC_MCT update", "TBMCTVERMAN update"}
  T13 = typedef "NI_Database_API.lvlib/Conn ObjectReference.ctl" = refnum<k1>
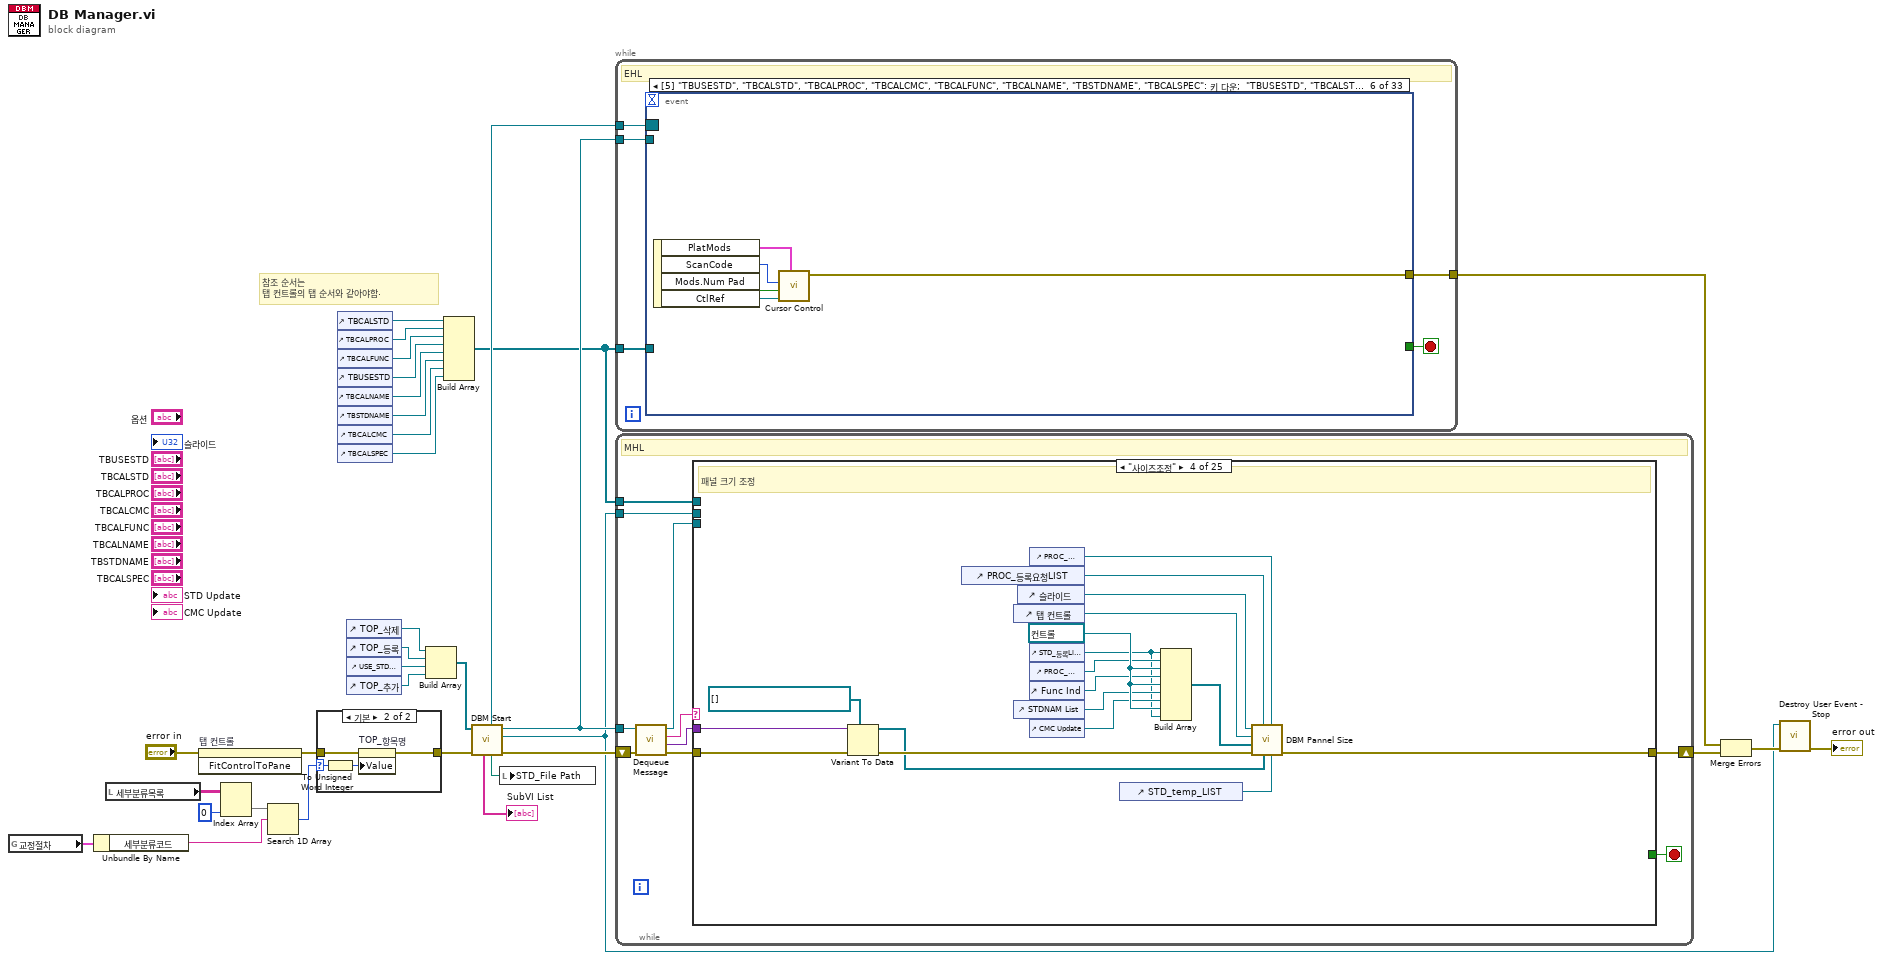
[diagram p0: block diagram]
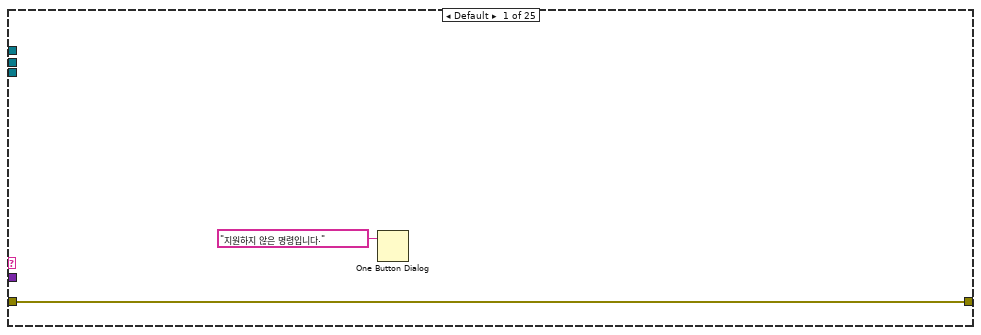
[diagram p3: hidden frame]
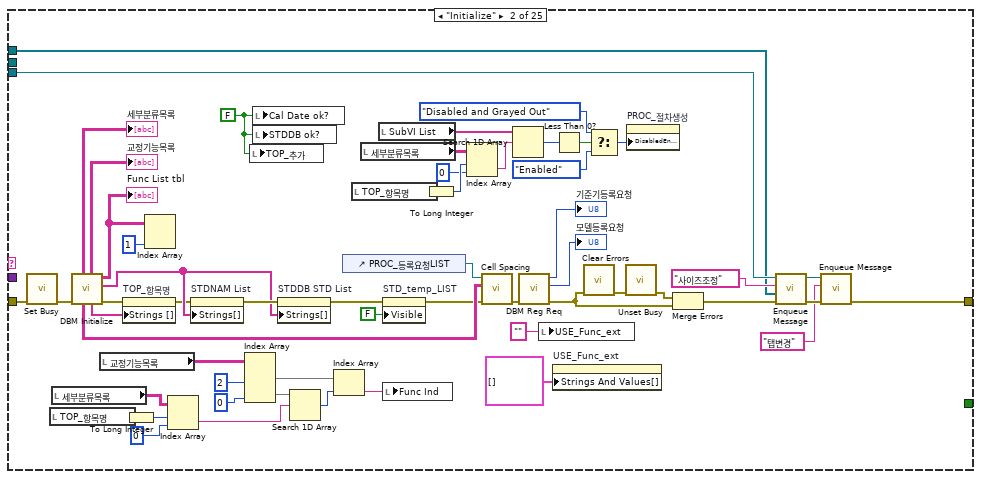
[diagram p4: hidden frame]
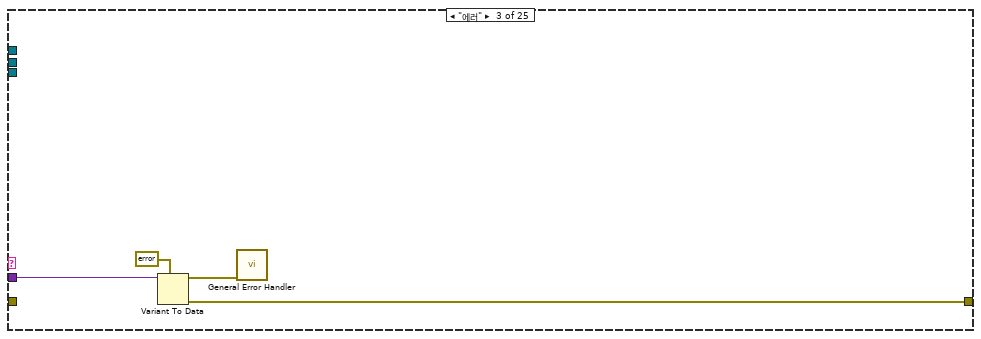
[diagram p5: hidden frame]
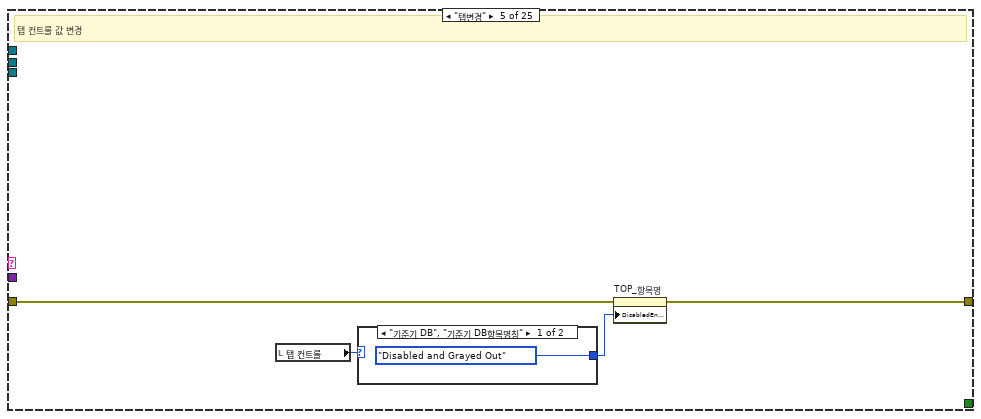
[diagram p6: hidden frame]
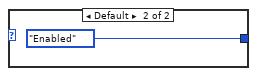
[diagram p7: hidden frame]
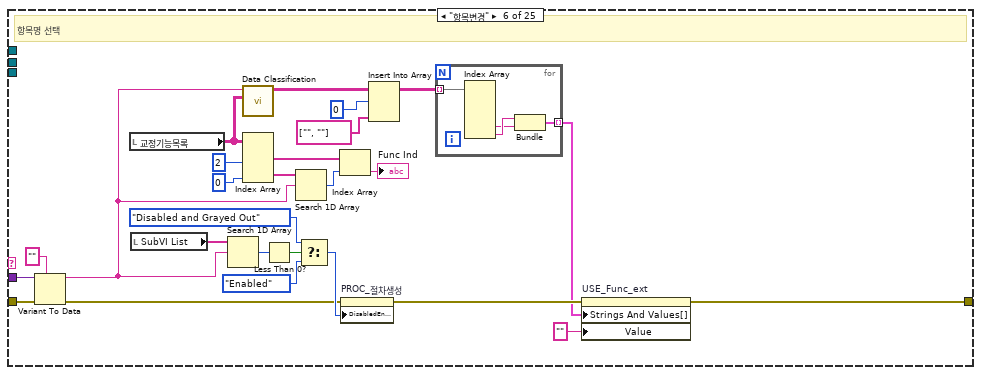
[diagram p8: hidden frame]
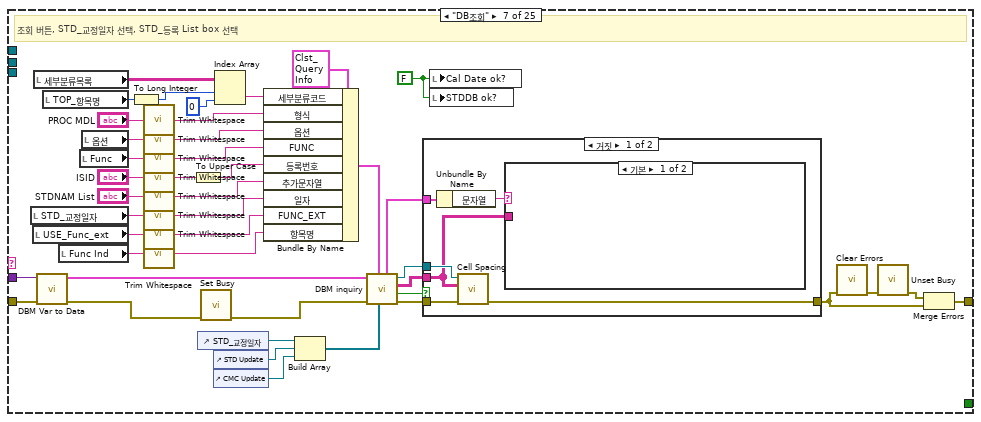
[diagram p9: hidden frame]
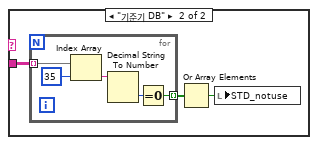
[diagram p10: hidden frame]
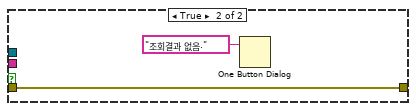
[diagram p11: hidden frame]
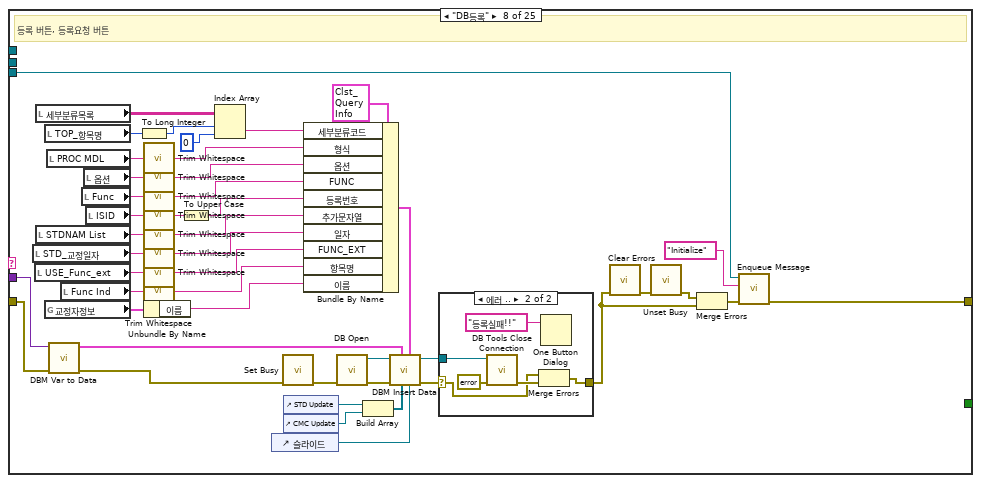
[diagram p12: hidden frame]
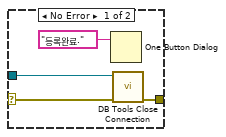
[diagram p13: hidden frame]
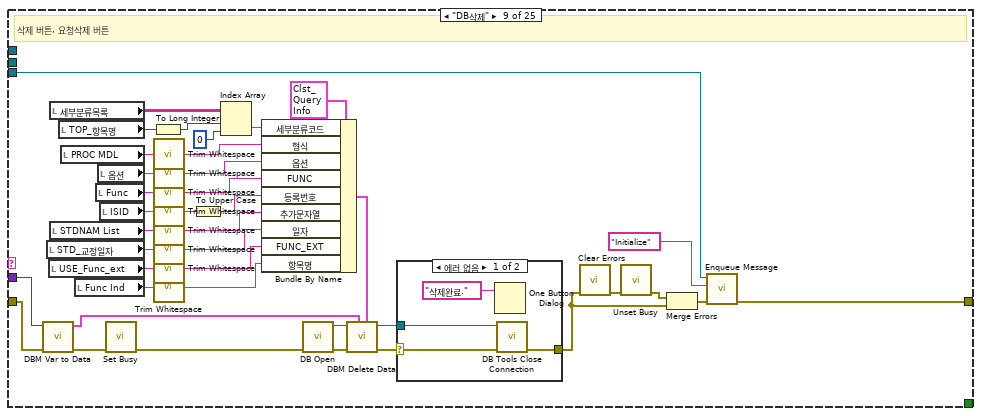
[diagram p14: hidden frame]
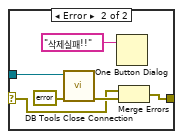
[diagram p15: hidden frame]
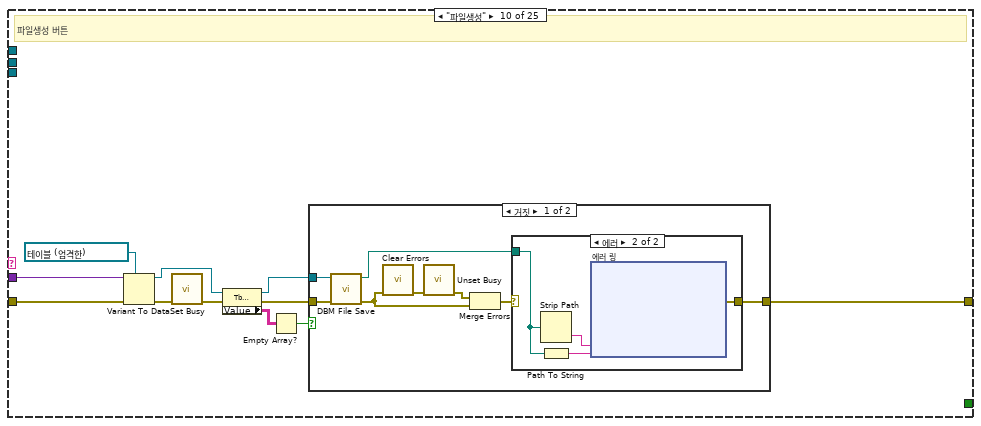
[diagram p16: hidden frame]
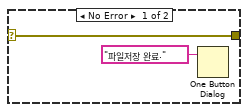
[diagram p17: hidden frame]
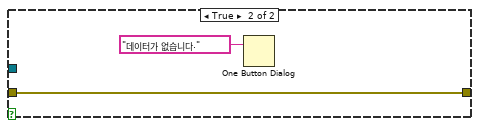
[diagram p18: hidden frame]
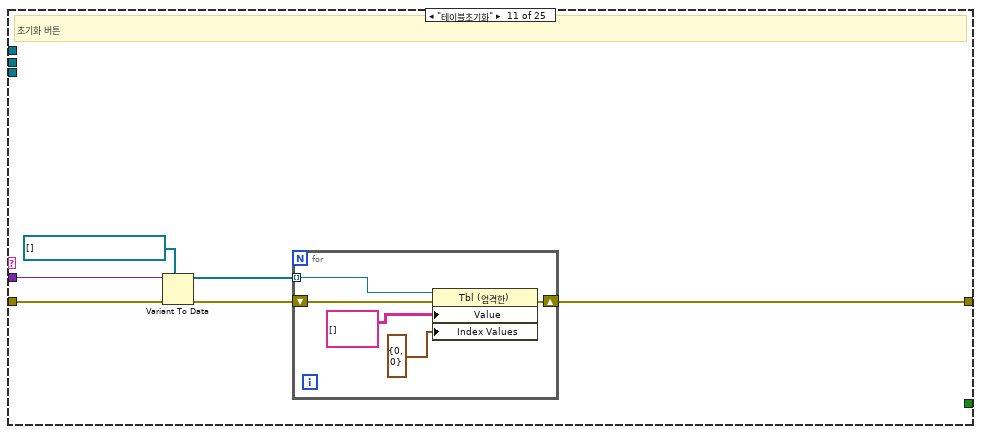
[diagram p19: hidden frame]
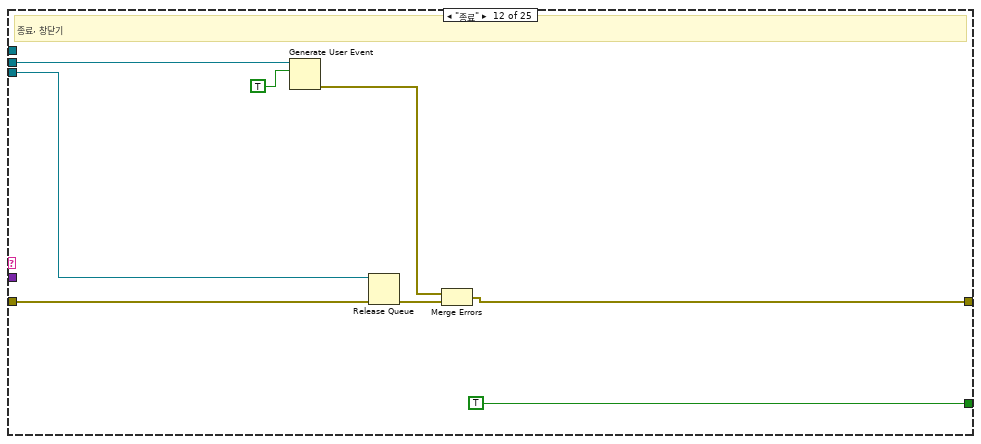
[diagram p20: hidden frame]
diagram:
  # "참조 순서는\n탭 컨트롤의 탭 순서와 같아야함."
  n1 = global read "Global_Cal Info.vi" "교정절차"() -> (w11:T2)
  n2 = Unbundle By Name(w11) -> ("세부분류코드"=w10:string)
  n3 = local read "세부분류목록"() -> (w7:string[][])
  n4 = invoke on="탭 컨트롤" class="TabCtl (엄격한)" method="FitControlToPane"(error in="error in") -> (error out=w8:errorcluster)  [unwired: 2 in, 2 out]
  n5 = Index Array(array=w7, index (col)=0 ("비활성화된 인덱스 (열)")) -> (element=w6:string[])  [unwired: 1 in]
  n6 = Search 1D Array(1D array=w6, element=w10) -> (index of element=w4:i32)  [unwired: 1 in]
  n7 = case shown="기본" w4 {
    selector: w4 -> [_ w36]
    tunnel: [w34 w38] -> w9
    tunnel: w8 -> [w34 w37]
    frame -1 {
    }
    frame Default {
      n8 = To Unsigned Word Integer(number=w36) -> (unsigned 16bit integer=w35:u16)
      n9 = property on="TOP_항목명" class="Ring (엄격한)"(error in=w37, "Value"=w35) -> (error out=w38:errorcluster)  [unwired: 1 in, 1 out]
    }
  }
  n10 = control-ref of="TBCALSTD"() -> (w2:refnum<vi>)
  n11 = control-ref of="TBCALPROC"() -> (w28:refnum<vi>)
  n12 = control-ref of="TBCALFUNC"() -> (w29:refnum<vi>)
  n13 = control-ref of="TBUSESTD"() -> (w12:refnum<vi>)
  n14 = control-ref of="TBCALNAME"() -> (w27:refnum<vi>)
  n15 = control-ref of="TBSTDNAME"() -> (w26:refnum<vi>)
  n16 = control-ref of="TBCALCMC"() -> (w24:refnum<vi>)
  n17 = control-ref of="TBCALSPEC"() -> (w22:refnum<vi>)
  n18 = control-ref of="TOP_삭제"() -> (w16:refnum<vi>)
  n19 = control-ref of="TOP_등록"() -> (w15:refnum<vi>)
  n20 = control-ref of="USE_STD 추가"() -> (w14:refnum<vi>)
  n21 = control-ref of="TOP_추가"() -> (w3:refnum<vi>)
  n22 = Build Array(w16, w15, w14, w3) -> (w13:refnum<vi>[])
  n23 = Build Array(w2, w28, w29, w12, w27, w26, w24, w22) -> (w1:refnum<vi>[])
  n24 = call "DBM Start.vi"("에러 입력(에러 없음)"=w9, "추가된 배열"=w13) -> ("에러 출력"=w23:errorcluster, "사용자 이벤트 - 정지"=w18:refnum<user-event>, "큐 출력"=w19:refnum<queue>, "dup path"=w20:path, "이벤트 등록 참조 번호 출력"=w17:refnum<event-registration>, "배열"=→"SubVI List":string[])  [unwired: 4 in]
  n25 = local write "STD_File Path"(w20) -> ()
  n26 = while {
    tunnel: [w43] -> w33
    tunnel: w19 -> [w42]
    tunnel: w17 -> [w41]
    tunnel: w1 -> [w39]
    stop <- w40 stop-if-true
    # "EHL"
    n27 = event shown="[5] \"TBUSESTD\", \"TBCALSTD\", \"TBCALPROC\", \"TBCALCMC\", \"TBCALFUNC\", \"TBCALNAME\", \"TBSTDNAME\", \"TBCALSPEC\": 키 다운;  \"TBUSESTD\", \"TBCALSTD\", \"TBCALPROC\", \"TBCALCMC\", \"TBCALFUNC\", \"TBCALNAME\", \"TBSTDNAME\", \"TBCALSPEC\": 키 반복" {
      selector: w41 -> [_ _ _ _ _ _ _ _ _ _ _ _ _ _ _ _ _ _ _ _ _ _ _ _ _ _ _ _ _ _ _ _ _]
      dyn-events: _ -> [_ _ _ _ _ _ _ _ _ _ _ _ _ _ _ _ _ _ _ _ _ _ _ _ _ _ _ _ _ _ _ _ _]
      timeout: _ -> [_ _ _ _ _ _ _ _ _ _ _ _ _ _ _ _ _ _ _ _ _ _ _ _ _ _ _ _ _ _ _ _ _]
      tunnel: [_ w49 w53 w57 w60 w63 w68 w77 w89 w96 w129 w163 w223 w269 w274 w278 w282 w298 w309 w317 w329 w338 w342 w351 w359 w375 w392 _ w401 w409 w411 w417 w425] -> w43
      tunnel: w42 -> [_ w48 w52 _ _ _ w67 w76 w88 w95 w128 w162 w222 w268 w273 w277 w283 w297 w308 w316 _ w339 w348 w350 w360 w376 w391 _ w400 w408 w410 w416 w426]
      tunnel: [w44 _ _ _ _ _ _ _ _ _ _ _ _ _ _ _ _ _ _ _ _ _ _ _ _ _ _ _ _ _ _ _ _] -> w40
      tunnel: w39 -> [_ _ w51 _ _ _ _ _ w83 _ _ w160 w219 w264 w271 _ _ _ _ _ _ _ _ _ _ _ _ _ _ _ _ _ _]
      event User Event {
        n28 = event-data() -> ("STOP"=w44:bool)  [unwired: 1 in]
      }
      event Panel Close? {
        n29 = event-data() -> ()  [unwired: 1 in, 1 out]
        n30 = call "Enqueue Message.vi"("우선순위 메시지?"=TRUE, "메세지"="종료", "큐 입력"=w48) -> ("에러 출력"=w49:errorcluster)  [unwired: 7 in, 1 out]
        n31 = event-data("Discard?"=TRUE ("버림?")) -> ()  [unwired: 1 in, 1 out]
      }
      event Panel Resize {
        n32 = event-data() -> ()  [unwired: 1 in, 1 out]
        n33 = To Variant(anything=w51) -> (Variant=w50:variant)
        n34 = call "Enqueue Message.vi"("값"=w50, "메세지"="사이즈조정", "큐 입력"=w52) -> ("에러 출력"=w53:errorcluster)  [unwired: 7 in, 1 out]
      }
      event "TBCALCMC", "TBCALPROC", "TBCALSTD", "TBUSESTD", "TBCALFUNC", "TBCALNAME", "TBSTDNAME", "TBCALSPEC": Shortcut Menu Selection (User) {
        n35 = event-data() -> ("CtlRef"=w56:refnum<vi>, "ItemTag"=w55:string)  [unwired: 1 in]
        n36 = call "Mouse PopUp Control.vi"("type"=Cmd_Mouse_Popup."메뉴선택", "아이템 태그"=w55, "Tbl 참조 번호"=w56) -> ("error out"=w57:errorcluster)  [unwired: 8 in]
      }
      event "TBCALCMC", "TBCALPROC", "TBCALSTD", "TBUSESTD", "TBCALFUNC", "TBCALNAME", "TBSTDNAME", "TBCALSPEC": Shortcut Menu Activation? {
        n37 = event-data() -> ("MenuRef"=w59:refnum<k9>)  [unwired: 1 in]
        n38 = call "Mouse PopUp Control.vi"("type"=Cmd_Mouse_Popup."활성화", "메뉴 참조"=w59) -> ("error out"=w60:errorcluster)  [unwired: 9 in]
        n39 = event-data() -> ()  [unwired: 2 in, 1 out]
      }
      event "TBUSESTD", "TBCALSTD", "TBCALPROC", "TBCALCMC", "TBCALFUNC", "TBCALNAME", "TBSTDNAME", "TBCALSPEC": Key Down; "TBUSESTD", "TBCALSTD", "TBCALPROC", "TBCALCMC", "TBCALFUNC", "TBCALNAME", "TBSTDNAME", "TBCALSPEC": Key Repeat {
        n40 = event-data() -> ("PlatMods"=w62:T5, "ScanCode"=w66:i16, "Mods.Num Pad"=w65:bool, "CtlRef"=w64:refnum<vi>)  [unwired: 1 in]
        n41 = call "Cursor Control.vi"("플랫폼 조합키"=w62, "참조"=w64, "Num Pad"=w65, "ScanCode"=w66) -> ("error out"=w63:errorcluster)  [unwired: 6 in, 1 out]
      }
      event "탭 컨트롤": Value Change {
        n42 = event-data() -> ()  [unwired: 1 in, 1 out]
        n43 = call "Enqueue Message.vi"("메세지"="탭변경", "큐 입력"=w67) -> ("에러 출력"=w68:errorcluster)  [unwired: 8 in, 1 out]
      }
      event "TOP_항목명": Value Change {
        n44 = event-data() -> ()  [unwired: 1 in, 2 out]
        n45 = local read "세부분류목록"() -> (w73:string[][])
        n46 = To Long Integer(number="TOP_항목명") -> (32bit integer=w75:i32)
        n47 = Index Array(array=w73, index (row)=w75, index (col)=0 ("비활성화된 인덱스 (열)")) -> (element=w72:string)
        n48 = To Variant(anything=w72) -> (Variant=w71:variant)
        n49 = call "Enqueue Message.vi"("값"=w71, "메세지"="항목변경", "큐 입력"=w76) -> ("에러 출력"=w77:errorcluster)  [unwired: 7 in, 1 out]
      }
      event "TOP_조회": Value Change {
        n50 = event-data() -> ()  [unwired: 1 in, 1 out]
        n51 = local read "탭 컨트롤"() -> (w84:T1)
        n52 = To Long Integer(number=w84) -> (32bit integer=w85:i32)
        n53 = Format Into String(w84) -> (resulting string=w81:string)  [unwired: 3 in, 1 out]
        n54 = Index Array(array=w83, index=w85) -> (element=w80:refnum<vi>)
        n55 = Bundle(cluster=T4 {"문자열"="", "불리언"=FALSE, "원소"=refnum} ("데이터"), "문자열"=w81, "원소"=w80) -> (w82:T4)  [unwired: 1 in]
        n56 = To Variant(anything=w82) -> (Variant=w86:variant)
        n57 = call "Enqueue Message.vi"("값"=w86, "메세지"="DB조회", "큐 입력"=w88) -> ("에러 출력"=w89:errorcluster)  [unwired: 7 in, 1 out]
      }
      event "TOP_등록요청": Value Change {
        n58 = event-data() -> ()  [unwired: 1 in, 1 out]
        n59 = local read "탭 컨트롤"() -> (w94:T1)
        n60 = case shown="\"교정절차 DB\"" w94 {
          tunnel: [_ "기준기등록요청" ("메세지") "절차복제" ("메세지")] -> w93
          tunnel: ["해당 기능 적용안됨." ("메시지") "등록번호 확인" ("메시지") "항목명을 선택하고 모델명을 입력하세요." ("메시지")] -> w92
          tunnel: [_ w102 w111] -> w91
          tunnel: [_ w100 w109] -> w90
          frame Default {
          }
          frame "기준기 DB" {
            n61 = local read "ISID"() -> (w99:string)
            n62 = call <vilib>:"Trim Whitespace.vi"("string"=w99) -> ("trimmed string"=w98:string)  [unwired: 1 in]
            n63 = control-ref of="TBCALSTD"() -> (w102:refnum<vi>)
            n64 = Empty String/Path?(string/path=w98) -> (empty?=w101:bool)
            n65 = Not(x=w101) -> (.not. x?=w100:bool)
          }
          frame "교정절차 DB" {
            n66 = local read "PROC MDL"() -> (w106:string)
            n67 = local read "TOP_항목명"() -> (w108:u16)
            n68 = Equal To 0?(x=w108) -> (x = 0?=w107:bool)
            n69 = call <vilib>:"Trim Whitespace.vi"("string"=w106) -> ("trimmed string"=w105:string)  [unwired: 1 in]
            n70 = control-ref of="TBCALPROC"() -> (w111:refnum<vi>)
            n71 = Empty String/Path?(string/path=w105) -> (empty?=w110:bool)
            n72 = Not Or(1:w110, 2:w107) -> (0:w109:bool)
          }
        }
        n73 = case shown="참" w90 {
          tunnel: [_ w122] -> w96
          tunnel: w95 -> [_ w121]
          tunnel: w93 -> [_ w117]
          tunnel: w92 -> [w114 _]
          tunnel: w91 -> [_ w115]
          frame False {
            n74 = One Button Dialog(message=w114) -> ()  [unwired: 1 in, 1 out]
          }
          frame True {
            n75 = Bundle(cluster=T4 {"문자열"="", "불리언"=FALSE, "원소"=refnum} ("데이터"), "문자열"=w117, "원소"=w115) -> (w119:T4)  [unwired: 1 in]
            n76 = To Variant(anything=w119) -> (Variant=w118:variant)
            n77 = call "Enqueue Message.vi"("값"=w118, "메세지"="DB등록", "큐 입력"=w121) -> ("에러 출력"=w122:errorcluster)  [unwired: 7 in, 1 out]
          }
        }
      }
      event "TOP_요청삭제": Value Change {
        n78 = event-data() -> ()  [unwired: 1 in, 1 out]
        n79 = local read "탭 컨트롤"() -> (w127:T1)
        n80 = Format Into String(w127) -> (resulting string=w126:string)  [unwired: 3 in, 1 out]
        n81 = case shown="\"교정절차 DB\"" w126 {
          tunnel: [_ "모델등록요청삭제" ("추가문자열") "기준기등록요청" ("추가문자열")] -> w125
          tunnel: [TRUE ("empty?") w132 w136] -> w124
          tunnel: [_ w131 w135] -> w123
          frame Default {
          }
          frame "교정절차 DB" {
            n82 = local read "TBCALPROC"() -> (w133:string[][])
            n83 = control-ref of="TBCALPROC"() -> (w131:refnum<vi>)
            n84 = Empty Array?(array=w133) -> (empty?=w132:bool)
          }
          frame "기준기 DB" {
            n85 = local read "TBCALSTD"() -> (w137:string[][])
            n86 = control-ref of="TBCALSTD"() -> (w135:refnum<vi>)
            n87 = Empty Array?(array=w137) -> (empty?=w136:bool)
          }
        }
        n88 = case shown="거짓" w124 {
          tunnel: [w146 _] -> w129
          tunnel: w128 -> [w145 _]
          tunnel: w125 -> [w141 _]
          tunnel: w123 -> [w139 _]
          frame False {
            n89 = Bundle(cluster=T4 {"문자열"="", "불리언"=FALSE, "원소"=refnum} ("데이터"), "문자열"=w141, "원소"=w139) -> (w143:T4)  [unwired: 1 in]
            n90 = To Variant(anything=w143) -> (Variant=w142:variant)
            n91 = call "Enqueue Message.vi"("값"=w142, "메세지"="DB삭제", "큐 입력"=w145) -> ("에러 출력"=w146:errorcluster)  [unwired: 7 in, 1 out]
          }
          frame True {
            n92 = One Button Dialog(message="삭제할 데이터가 없습니다." ("메시지")) -> ()  [unwired: 1 in, 1 out]
          }
        }
      }
      event "TOP_등록", "TOP_추가": Value Change {
        n93 = event-data() -> ()  [unwired: 1 in, 1 out]
        n94 = local read "세부분류목록"() -> (w153:string[][])
        n95 = local read "탭 컨트롤"() -> (w152:T1)
        n96 = local read "TOP_항목명"() -> (w156:u16)
        n97 = To Long Integer(number=w152) -> (32bit integer=w161:i32)
        n98 = To Long Integer(number=w156) -> (32bit integer=w154:i32)
        n99 = Format Into String(w152) -> (resulting string=w158:string)  [unwired: 3 in, 1 out]
        n100 = Index Array(array=w160, index=w161) -> (element=w159:refnum<vi>)
        n101 = Index Array(array=w153, index (row)=w154, index (col)=0 ("비활성화된 인덱스 (열)")) -> (element=w151:string)
        n102 = property class="Tbl (엄격한)"(reference=w159) -> (reference out=w148:refnum<vi>, "Value"=w150:string[][])  [unwired: 1 in, 1 out]
        n103 = case shown="\"기준기 DB\"" w152 {
          tunnel: [_ w187 w191 w197 w203] -> w157
          tunnel: w150 -> [_ _ w195 w201 w207]
          tunnel: w151 -> [_ _ w190 w196 w202]
          frame Default {
          }
          frame "기준기 DB" {
            n104 = local read "Cal Date ok?"() -> (w189:bool)
            n105 = local read "STDDB ok?"() -> (w188:bool)
            n106 = Not And(1:w188, 2:w189) -> (0:w187:bool)
          }
          frame "교정절차 DB", "CMC DB" {
            n107 = Index Array(array=w195, index (row)=0 ("인덱스 (행)"), index (col)=2 ("비활성화된 인덱스 (열)")) -> (element=w192:string)
            n108 = Not Equal?(x=w190, y=w192) -> (x != y?=w191:bool)
          }
          frame "교정절차항목명칭", "SPEC DB" {
            n109 = Index Array(array=w201, index (row)=0 ("인덱스 (행)"), index (col)=1 ("비활성화된 인덱스 (열)")) -> (element=w198:string)
            n110 = Not Equal?(x=w196, y=w198) -> (x != y?=w197:bool)
          }
          frame "교정기능 DB" {
            n111 = Index Array(array=w207, index (row)=0 ("인덱스 (행)"), index (col)=0 ("비활성화된 인덱스 (열)")) -> (element=w204:string)
            n112 = Not Equal?(x=w202, y=w204) -> (x != y?=w203:bool)
          }
        }
        n113 = Empty Array?(array=w150) -> (empty?=w149:bool)
        n114 = case shown="거짓" w149 {
          tunnel: [w168 _] -> w163
          tunnel: w162 -> [w167 _]
          tunnel: w158 -> [w166 _]
          tunnel: w157 -> [w165 _]
          tunnel: w148 -> [w164 _]
          frame False {
            n115 = case shown="거짓" w165 {
              tunnel: [w177 _] -> w168
              tunnel: w167 -> [w176 _]
              tunnel: w166 -> [w173 w183]
              tunnel: w164 -> [w169 _]
              frame False {
                n116 = Bundle(cluster=T4 {"문자열"="", "불리언"=FALSE, "원소"=refnum} ("데이터"), "문자열"=w173, "불리언"="TOP_추가", "원소"=w169) -> (w172:T4)
                n117 = Two Button Dialog(message="화면에 보이는 내용으로 업데이트 됩니다.\n해당 내용은 복구가 불가능 합니다.\n계속하시겠습니까?" ("메시지")) -> (T button?=w175:bool)  [unwired: 2 in]
                n118 = case shown="참" w175 {
                  tunnel: [_ w182] -> w177
                  tunnel: w176 -> [_ w181]
                  tunnel: w172 -> [_ w178]
                  frame False {
                  }
                  frame True {
                    n119 = To Variant(anything=w178) -> (Variant=w179:variant)
                    n120 = call "Enqueue Message.vi"("값"=w179, "메세지"="DB등록", "큐 입력"=w181) -> ("에러 출력"=w182:errorcluster)  [unwired: 7 in, 1 out]
                  }
                }
              }
              frame True {
                n121 = case shown="\"기준기 DB\"" w183 {
                  frame Default {
                    n122 = One Button Dialog(message="데이터 또는 항목명에 오류가 있습니다." ("메시지")) -> ()  [unwired: 1 in, 1 out]
                  }
                  frame "기준기 DB" {
                    n123 = One Button Dialog(message="교정일자일치 여부, 등록 가능 여부 확인." ("메시지")) -> ()  [unwired: 1 in, 1 out]
                  }
                }
              }
            }
          }
          frame True {
            n124 = One Button Dialog(message="등록 할 데이터가 없습니다." ("메시지")) -> ()  [unwired: 1 in, 1 out]
          }
        }
      }
      event "TOP_삭제": Value Change {
        n125 = event-data() -> ()  [unwired: 1 in, 1 out]
        n126 = local read "세부분류목록"() -> (w212:string[][])
        n127 = local read "탭 컨트롤"() -> (w211:T1)
        n128 = local read "TOP_항목명"() -> (w215:u16)
        n129 = To Long Integer(number=w215) -> (32bit integer=w213:i32)
        n130 = To Long Integer(number=w211) -> (32bit integer=w220:i32)
        n131 = Format Into String(w211) -> (resulting string=w216:string)  [unwired: 3 in, 1 out]
        n132 = Index Array(array=w219, index=w220) -> (element=w218:refnum<vi>)
        n133 = Index Array(array=w212, index (row)=w213, index (col)=0 ("비활성화된 인덱스 (열)")) -> (element=w208:string)
        n134 = property class="Tbl (엄격한)"(reference=w218) -> (reference out=w217:refnum<vi>, "Value"=w210:string[][])  [unwired: 1 in, 1 out]
        n135 = case shown="\"교정절차 DB\", \"CMC DB\"" w211 {
          tunnel: w210 -> [_ w246 w252 w258]
          tunnel: [_ w245 w251 w257] -> w209
          tunnel: w208 -> [_ w244 w250 w256]
          frame Default {
          }
          frame "교정절차 DB", "CMC DB" {
            n136 = Index Array(array=w246, index (row)=0 ("인덱스 (행)"), index (col)=2 ("비활성화된 인덱스 (열)")) -> (element=w247:string)
            n137 = Not Equal?(x=w244, y=w247) -> (x != y?=w245:bool)
          }
          frame "교정기능 DB" {
            n138 = Index Array(array=w252, index (row)=0 ("인덱스 (행)"), index (col)=0 ("비활성화된 인덱스 (열)")) -> (element=w253:string)
            n139 = Not Equal?(x=w250, y=w253) -> (x != y?=w251:bool)
          }
          frame "교정절차항목명칭", "SPEC DB" {
            n140 = Index Array(array=w258, index (row)=0 ("인덱스 (행)"), index (col)=1 ("비활성화된 인덱스 (열)")) -> (element=w259:string)
            n141 = Not Equal?(x=w256, y=w259) -> (x != y?=w257:bool)
          }
        }
        n142 = Empty Array?(array=w210) -> (empty?=w221:bool)
        n143 = case shown="거짓" w209 {
          tunnel: [w228 _] -> w223
          tunnel: w222 -> [w227 _]
          tunnel: w221 -> [w226 _]
          tunnel: w217 -> [w225 _]
          tunnel: w216 -> [w224 _]
          frame False {
            n144 = case shown="거짓" w226 {
              tunnel: [w236 _] -> w228
              tunnel: w227 -> [w235 _]
              tunnel: w224 -> [w231 _]
              tunnel: w225 -> [w230 _]
              frame False {
                n145 = Bundle(cluster=T4 {"문자열"="", "불리언"=FALSE, "원소"=refnum} ("데이터"), "문자열"=w231, "원소"=w230) -> (w229:T4)  [unwired: 1 in]
                n146 = Two Button Dialog(message="삭제후 복구가 불가능합니다.\n삭제하시겠습니까?" ("메시지")) -> (T button?=w234:bool)  [unwired: 2 in]
                n147 = case shown="참" w234 {
                  tunnel: [_ w241] -> w236
                  tunnel: w235 -> [_ w240]
                  tunnel: w229 -> [_ w237]
                  frame False {
                  }
                  frame True {
                    n148 = To Variant(anything=w237) -> (Variant=w238:variant)
                    n149 = call "Enqueue Message.vi"("값"=w238, "메세지"="DB삭제", "큐 입력"=w240) -> ("에러 출력"=w241:errorcluster)  [unwired: 7 in, 1 out]
                  }
                }
              }
              frame True {
                n150 = One Button Dialog(message="삭제 할 데이터가 없습니다." ("메시지")) -> ()  [unwired: 1 in, 1 out]
              }
            }
          }
          frame True {
            n151 = One Button Dialog(message="데이터 또는 항목명에 오류가 있습니다." ("메시지")) -> ()  [unwired: 1 in, 1 out]
          }
        }
      }
      event "TOP_파일생성": Value Change {
        n152 = event-data() -> ()  [unwired: 1 in, 1 out]
        n153 = local read "탭 컨트롤"() -> (w266:T1)
        n154 = To Long Integer(number=w266) -> (32bit integer=w265:i32)
        n155 = Index Array(array=w264, index=w265) -> (element=w263:refnum<vi>)
        n156 = To Variant(anything=w263) -> (Variant=w262:variant)
        n157 = call "Enqueue Message.vi"("값"=w262, "메세지"="파일생성", "큐 입력"=w268) -> ("에러 출력"=w269:errorcluster)  [unwired: 7 in, 1 out]
      }
      event "TOP_초기화": Value Change {
        n158 = event-data() -> ()  [unwired: 1 in, 1 out]
        n159 = To Variant(anything=w271) -> (Variant=w270:variant)
        n160 = call "Enqueue Message.vi"("값"=w270, "메세지"="테이블초기화", "큐 입력"=w273) -> ("에러 출력"=w274:errorcluster)  [unwired: 7 in, 1 out]
      }
      event "TOP_종료": Value Change {
        n161 = event-data() -> ()  [unwired: 1 in, 1 out]
        n162 = call "Enqueue Message.vi"("우선순위 메시지?"=TRUE, "메세지"="종료", "큐 입력"=w277) -> ("에러 출력"=w278:errorcluster)  [unwired: 7 in, 1 out]
      }
      event "STD_교정일자": Value Change {
        n163 = event-data() -> ()  [unwired: 1 in, 1 out]
        n164 = call <vilib>:"Trim Whitespace.vi"("string"="STD_교정일자") -> ("trimmed string"=w280:string)  [unwired: 1 in]
        n165 = Empty String/Path?(string/path=w280) -> (empty?=w281:bool)
        n166 = case shown="거짓" w281 {
          tunnel: w283 -> [w291 _]
          tunnel: [w290 _] -> w282
          frame False {
            n167 = control-ref of="TBCALSTD"() -> (w284:refnum<vi>)
            n168 = Bundle(cluster=T4 {"문자열"="", "불리언"=FALSE, "원소"=refnum} ("데이터"), "문자열"="기준기 DB_BACK" ("메세지"), "원소"=w284) -> (w287:T4)  [unwired: 1 in]
            n169 = To Variant(anything=w287) -> (Variant=w288:variant)
            n170 = call "Enqueue Message.vi"("값"=w288, "메세지"="DB조회", "큐 입력"=w291) -> ("에러 출력"=w290:errorcluster)  [unwired: 7 in, 1 out]
          }
          frame True {
            n171 = One Button Dialog(message="교정일자를 선택하세요." ("메시지")) -> ()  [unwired: 1 in, 1 out]
          }
        }
      }
      event "STD_File Path", "STD_다시열기": Value Change {
        n172 = event-data() -> ()  [unwired: 1 in, 2 out]
        n173 = call <vilib>:"Get File Extension.vi"("file"="STD_File Path") -> ("error out"=w294:errorcluster, "lowercase file extension"=w293:string, "dup file"=w295:path)  [unwired: 6 in, 2 out]
        n174 = case shown="기본" w293 {
          tunnel: [w300 w306] -> w298
          tunnel: w297 -> [_ w305]
          tunnel: w295 -> [_ w303]
          tunnel: w294 -> [w300 w302]
          frame "" {
            n175 = One Button Dialog(message="파일명이 잘못되었음." ("메시지")) -> ()  [unwired: 1 in, 1 out]
          }
          frame Default {
            n176 = To Variant(anything=w303) -> (Variant=w301:variant)
            n177 = call "Enqueue Message.vi"("에러 입력(에러 없음)"=w302, "값"=w301, "메세지"="기준기성적서파일열기", "큐 입력"=w305) -> ("에러 출력"=w306:errorcluster)  [unwired: 6 in, 1 out]
          }
        }
      }
      event "STD_등록List 검색": Value Change {
        n178 = event-data() -> ()  [unwired: 1 in, 1 out]
        n179 = call "Enqueue Message.vi"("메세지"="기준기등록리스트검색", "큐 입력"=w308) -> ("에러 출력"=w309:errorcluster)  [unwired: 8 in, 1 out]
      }
      event "STD_List box": Double Click {
        n180 = event-data() -> ()  [unwired: 1 in, 1 out]
        n181 = property on="STD_List box" class="MCListbox (엄격한)"("Visible"=FALSE ("보이기")) -> (error out=w315:errorcluster, "ItemNames"=w314:string[][])  [unwired: 2 in, 1 out]
        n182 = Index Array(array=w314, index (row)="STD_List box", index (col)=0 ("비활성화된 인덱스 (열)")) -> (element=w313:string)
        n183 = case shown="기본" w313 {
          selector: w313 -> [_ w321]
          tunnel: [w318 w325] -> w317
          tunnel: w316 -> [_ w324]
          tunnel: w315 -> [w318 w323]
          frame "" {
          }
          frame Default {
            n184 = local write "ISID"(w321) -> ()
            n185 = control-ref of="TBCALSTD"() -> (w319:refnum<vi>)
            n186 = Bundle(cluster=T4 {"문자열"="", "불리언"=FALSE, "원소"=refnum} ("데이터"), "문자열"="기준기 DB" ("메세지"), "원소"=w319) -> (w326:T4)  [unwired: 1 in]
            n187 = To Variant(anything=w326) -> (Variant=w327:variant)
            n188 = call "Enqueue Message.vi"("에러 입력(에러 없음)"=w323, "값"=w327, "메세지"="DB조회", "큐 입력"=w324) -> ("에러 출력"=w325:errorcluster)  [unwired: 6 in, 1 out]
          }
        }
      }
      event "STD_DB오류목록": Value Change {
        n189 = event-data() -> ()  [unwired: 1 in, 2 out]
        n190 = call "STD Cal Date Check.vi"() -> ("error out"=w331:errorcluster, "비어있음?"=w332:bool, "Data"=w330:string[][])  [unwired: 9 in]
        n191 = case shown="거짓" w332 {
          tunnel: w331 -> [w335 w337]
          tunnel: [w334 w337] -> w329
          tunnel: w330 -> [w333 _]
          frame False {
            n192 = call "View STD Error.vi"("error in"=w335, "Data"=w333) -> ("error out"=w334:errorcluster)  [unwired: 9 in]
          }
          frame True {
            n193 = One Button Dialog(message="오류가 없습니다." ("메시지")) -> ()  [unwired: 1 in, 1 out]
          }
        }
      }
      event "STD_DB요청리스트": Value Change {
        n194 = event-data() -> ()  [unwired: 1 in, 2 out]
        n195 = call "Enqueue Message.vi"("메세지"="기준기DB요청열기", "큐 입력"=w339) -> ("에러 출력"=w338:errorcluster)  [unwired: 8 in, 1 out]
      }
      event "STD_temp_LIST": Double Click {
        n196 = event-data() -> ()  [unwired: 1 in, 2 out]
        n197 = To Variant(anything="STD_temp_LIST") -> (Variant=w346:variant)
        n198 = call "Enqueue Message.vi"("값"=w346, "메세지"="기준기DB요청선택", "큐 입력"=w348) -> ("에러 출력"=w343:errorcluster, "큐 출력"=w341:refnum<queue>)  [unwired: 7 in]
        n199 = call "Enqueue Message.vi"("에러 입력(에러 없음)"=w343, "메세지"="기준기교정값내용검토", "큐 입력"=w341) -> ("에러 출력"=w342:errorcluster)  [unwired: 7 in, 1 out]
      }
      event "STD_DB 내용 검토": Value Change {
        n200 = event-data() -> ()  [unwired: 1 in, 1 out]
        n201 = call "Enqueue Message.vi"("메세지"="기준기교정값내용검토", "큐 입력"=w350) -> ("에러 출력"=w351:errorcluster)  [unwired: 8 in, 1 out]
      }
      event "STD_notuse": Value Change {
        n202 = event-data() -> ()  [unwired: 1 in, 2 out]
        n203 = Not(x="STD_notuse") -> (.not. x?=w362:bool)
        n204 = Boolean To (0,1)(Boolean=w362) -> (0, 1=w354:i16)
        n205 = local read "TBCALSTD"() -> (w365:string[][])
        n206 = Format Into String(w354) -> (resulting string=w353:string, error out=w357:errorcluster)  [unwired: 3 in]
        n207 = for {
          tunnel: w365 -> [w370] mode=indexing
          tunnel: w353 -> [w368]
          tunnel: [w367] -> w363 mode=indexing
          shift-right: [w366] -> w356
          shift-left: w357 -> [w366]
          n208 = Replace Array Subset(array=w370, new element=w368, index=35 ("인덱스")) -> (w367:string[])
        }
        n209 = local write "TBCALSTD"(w363) -> ()
        n210 = Bundle(cluster=T4 {"문자열"="", "불리언"=FALSE, "원소"=refnum} ("데이터"), "문자열"=w353) -> (w355:T4)  [unwired: 2 in]
        n211 = To Variant(anything=w355) -> (Variant=w358:variant)
        n212 = call "Enqueue Message.vi"("에러 입력(에러 없음)"=w356, "값"=w358, "메세지"="DB업데이트", "큐 입력"=w360) -> ("에러 출력"=w359:errorcluster)  [unwired: 6 in, 1 out]
      }
      event "PROC_모델 선택": Value Change {
        n213 = event-data() -> ()  [unwired: 1 in, 1 out]
        n214 = control-ref of="TBCALPROC"() -> (w374:refnum<vi>)
        n215 = call <vilib>:"Trim Whitespace.vi"("string"="PROC_모델 선택") -> ("trimmed string"=w372:string)  [unwired: 1 in]
        n216 = case shown="기본" w372 {
          tunnel: w376 -> [_ w383]
          tunnel: [_ w382] -> w375
          tunnel: "교정절차 DB" ("메세지") -> [_ w379]
          tunnel: w374 -> [_ w377]
          frame "" {
          }
          frame Default {
            n217 = Bundle(cluster=T4 {"문자열"="", "불리언"=FALSE, "원소"=refnum} ("데이터"), "문자열"=w379, "원소"=w377) -> (w381:T4)  [unwired: 1 in]
            n218 = To Variant(anything=w381) -> (Variant=w380:variant)
            n219 = call "Enqueue Message.vi"("값"=w380, "메세지"="모델선택", "큐 입력"=w383) -> ("에러 출력"=w382:errorcluster)  [unwired: 7 in, 1 out]
          }
        }
      }
      event "PROC_절차생성": Value Change {
        n220 = event-data() -> ()  [unwired: 1 in, 1 out]
        n221 = local read "TOP_항목명"() -> (w390:u16)
        n222 = local read "세부분류목록"() -> (w387:string[][])
        n223 = To Long Integer(number=w390) -> (32bit integer=w389:i32)
        n224 = Index Array(array=w387, index (row)=w389, index (col)=0 ("비활성화된 인덱스 (열)")) -> (element=w386:string)
        n225 = To Variant(anything=w386) -> (Variant=w385:variant)
        n226 = call "Enqueue Message.vi"("값"=w385, "메세지"="절차생성", "큐 입력"=w391) -> ("에러 출력"=w392:errorcluster)  [unwired: 7 in, 1 out]
      }
      event "PROC_지우기 1", "PROC_지우기 2": Value Change {
        n227 = event-data() -> ("CtlRef"=w395:refnum<vi>)  [unwired: 1 in]
        n228 = control-ref of="PROC_지우기 1"() -> (w396:refnum<vi>)
        n229 = Equal?(x=w396, y=w395) -> (x = y?=w394:bool)
        n230 = case shown="참" w394 {
          frame False {
            n231 = local write "옵션"("" ("PROC MDL")) -> ()
          }
          frame True {
            w398 = "" ("PROC MDL")
            n232 = local write "PROC MDL"(w398) -> ()
            n233 = local write "옵션"(w398) -> ()
          }
        }
      }
      event "PROC_모델 검색": Value Change {
        n234 = event-data() -> ()  [unwired: 1 in, 1 out]
        n235 = call "Enqueue Message.vi"("메세지"="모델검색", "큐 입력"=w400) -> ("에러 출력"=w401:errorcluster)  [unwired: 8 in, 1 out]
      }
      event "PROC_등록요청LIST": Double Click {
        n236 = event-data() -> ()  [unwired: 1 in, 1 out]
        n237 = property on="PROC_등록요청LIST" class="MCListbox (엄격한)"() -> (error out=w406:errorcluster, "ItemNames"=w405:string[][])  [unwired: 2 in, 1 out]
        n238 = Index Array(array=w405, index (row)="PROC_등록요청LIST") -> (element=w402:string[])  [unwired: 1 in]
        n239 = To Variant(anything=w402) -> (Variant=w403:variant)
        n240 = call "Enqueue Message.vi"("에러 입력(에러 없음)"=w406, "값"=w403, "메세지"="등록요청내용 조회", "큐 입력"=w408) -> ("에러 출력"=w409:errorcluster)  [unwired: 6 in, 1 out]
      }
      event "PROC_새로고침": Value Change {
        n241 = event-data() -> ()  [unwired: 1 in, 1 out]
        n242 = call "Enqueue Message.vi"("메세지"="등록요청리스트 갱신", "큐 입력"=w410) -> ("에러 출력"=w411:errorcluster)  [unwired: 8 in, 1 out]
      }
      event "USE_Func_ext": Value Change {
        n243 = event-data() -> ()  [unwired: 1 in, 1 out]
        n244 = To Variant(anything="USE_Func_ext") -> (Variant=w413:variant)
        n245 = call "Enqueue Message.vi"("값"=w413, "메세지"="세부교정기능목록", "큐 입력"=w416) -> ("에러 출력"=w417:errorcluster)  [unwired: 7 in, 1 out]
      }
      event "USE_STD 추가": Value Change {
        n246 = event-data() -> ()  [unwired: 1 in, 1 out]
        n247 = local read "USE_Func_ext"() -> (w420:string)
        n248 = local read "Func"() -> (w419:string)
        n249 = call <vilib>:"Trim Whitespace.vi"("string"=w419) -> ("trimmed string"=w423:string)  [unwired: 1 in]
        n250 = call <vilib>:"Trim Whitespace.vi"("string"=w420) -> ("trimmed string"=w424:string)  [unwired: 1 in]
        n251 = Empty String/Path?(string/path=w423) -> (empty?=w422:bool)
        n252 = Empty String/Path?(string/path=w424) -> (empty?=w421:bool)
        n253 = Or(x=w422, y=w421) -> (x .or. y?=w418:bool)
        n254 = case shown="거짓" w418 {
          tunnel: w426 -> [w434 _]
          tunnel: [w433 _] -> w425
          frame False {
            n255 = local read "TOP_항목명"() -> (w429:u16)
            n256 = local read "세부분류목록"() -> (w430:string[][])
            n257 = Index Array(array=w430, index (row)=w429, index (col)=0 ("비활성화된 인덱스 (열)")) -> (element=w428:string)
            n258 = To Variant(anything=w428) -> (Variant=w427:variant)
            n259 = call "Enqueue Message.vi"("값"=w427, "메세지"="사용기준기추가", "큐 입력"=w434) -> ("에러 출력"=w433:errorcluster)  [unwired: 7 in, 1 out]
          }
          frame True {
            n260 = One Button Dialog(message="교정속성목록 또는 세부교정속성이\n선택되지 않았습니다." ("메시지")) -> ()  [unwired: 1 in, 1 out]
          }
        }
      }
    }
  }
  n261 = while {
    shift-right: [w439] -> w30
    shift-left: w23 -> [w445]
    tunnel: w19 -> [w444]
    tunnel: w18 -> [w437]
    tunnel: w1 -> [w436]
    stop <- w438 stop-if-true
    # "MHL"
    n262 = call "Dequeue Message.vi"("에러 입력(에러 없음)"=w445, "큐 입력"=w444) -> ("에러 출력"=w443:errorcluster, "값"=w442:variant, "메세지"=w441:string, "큐 출력"=w440:refnum<queue>)  [unwired: 6 in]
    n263 = case shown="\"사이즈조정\"" w441 {
      tunnel: w443 -> [w447 w503 _ w512 w528 w536 w570 w625 w716 w731 w765 w778 w785 w865 w873 w897 w937 w973 w1005 w1025 w1039 w1125 w1148 w1166 w1208]
      tunnel: w442 -> [_ _ w504 w510 _ w535 w571 w623 w715 w730 w764 _ w783 _ _ w895 _ w971 w1004 w1026 _ w1124 _ w1165 w1207]
      tunnel: w440 -> [_ w478 _ _ _ _ _ w665 w706 _ _ w773 _ _ _ _ _ w977 w1008 _ _ _ _ _ _]
      tunnel: [w447 w468 w505 w516 w527 w548 w602 w666 w707 w736 w761 w777 w802 w860 w872 w898 w932 w978 w1009 w1028 w1064 w1110 w1149 w1167 w1213] -> w439
      tunnel: [_ _ _ _ _ _ _ _ _ _ _ TRUE _ _ _ _ _ _ _ _ _ _ _ _ _] -> w438
      tunnel: w437 -> [_ _ _ _ _ _ _ _ _ _ _ w774 _ _ _ _ _ _ _ _ _ _ _ _ _]
      tunnel: w436 -> [_ w448 _ _ _ _ _ _ _ _ _ _ _ _ _ _ _ _ _ _ _ _ _ _ _]
      frame Default {
        n264 = One Button Dialog(message="지원하지 않은 명령입니다." ("메시지")) -> ()  [unwired: 1 in, 1 out]
      }
      frame "Initialize" {
        w449 = FALSE ("Cal Date ok?")
        n265 = call <vilib>:"Set Busy.vi"("error in (no error)"=w503) -> ("error out"=w474:errorcluster)  [unwired: 9 in, 1 out]
        n266 = local read "TOP_항목명"() -> (w453:u16)
        n267 = local read "세부분류목록"() -> (w456:string[][])
        n268 = call "DBM Initialize.vi"("에러 입력"=w474) -> ("에러 출력"=w500:errorcluster, "STD List"=w485:string[], "Func List"=w484:string[][], "항목명"=w477:string[], "교정기능목록"=→"교정기능목록":string[][], "모델요청 List"=w481:string[][], "세부분류목록"=→"세부분류목록":string[][])  [unwired: 4 in]
        "Func List tbl" <- w484
        n269 = local read "교정기능목록"() -> (w451:string[][])
        n270 = property on="TOP_항목명" class="Ring (엄격한)"(error in=w500, "Strings []"=w477) -> (error out=w465:errorcluster)  [unwired: 1 in, 1 out]
        n271 = To Long Integer(number=w453) -> (32bit integer=w454:i32)
        n272 = Index Array(array=w484, index (col)=1 ("비활성화된 인덱스 (열)")) -> ()  [unwired: 1 in, 1 out]
        n273 = Index Array(array=w456, index (row)=w454, index (col)=0 ("비활성화된 인덱스 (열)")) -> (element=w452:string)
        n274 = property on="STDNAM List" class="CmbBox"(error in=w465, "Strings[]"=w485) -> (error out=w497:errorcluster)  [unwired: 1 in, 1 out]
        n275 = Index Array(array=w451, index (col) #1=2 ("비활성화된 인덱스 (열)"), index (col) #2=0 ("비활성화된 인덱스 (열)")) -> (element #1=w461:string[], element #2=w460:string[])  [unwired: 2 in]
        n276 = local write "TOP_추가"(w449) -> ()
        n277 = local write "Cal Date ok?"(w449) -> ()
        n278 = local write "STDDB ok?"(w449) -> ()
        n279 = property on="STDDB STD List" class="CmbBox"(error in=w497, "Strings[]"=w485) -> (error out=w464:errorcluster)  [unwired: 1 in, 1 out]
        n280 = Search 1D Array(1D array=w460, element=w452) -> (index of element=w459:i32)  [unwired: 1 in]
        n281 = Index Array(array=w461, index=w459) -> (element=w462:string)
        n282 = control-ref of="PROC_등록요청LIST"() -> (w482:refnum<vi>)
        n283 = local read "TOP_항목명"() -> (w486:u16)
        n284 = local read "세부분류목록"() -> (w489:string[][])
        n285 = local read "SubVI List"() -> (w490:string[])
        n286 = property on="STD_temp_LIST" class="MCListbox (엄격한)"(error in=w464, "Visible"=FALSE ("보이기")) -> (error out=w476:errorcluster)  [unwired: 1 in, 1 out]
        n287 = local write "Func Ind"(w462) -> ()
        n288 = To Long Integer(number=w486) -> (32bit integer=w488:i32)
        n289 = Index Array(array=w489, index (row)=w488, index (col)=0 ("비활성화된 인덱스 (열)")) -> (element=w496:string)
        n290 = call-poly "Cell Spacing.vi"("error in"=w476, "Data in"=w481, "여러열리스트박스 참조 in"=w482) -> ("error out"=w473:errorcluster)  [unwired: 7 in, 1 out]
        n291 = Search 1D Array(1D array=w490, element=w496) -> (index of element=w491:i32)  [unwired: 1 in]
        n292 = call "DBM Reg Req.vi"("에러 입력(에러 없음)"=w473) -> ("에러 출력"=w472:errorcluster, "모델 요청 갯수"=→"모델등록요청":u8, "기준기 요청 갯수"=→"기준기등록요청":u8)  [unwired: 6 in, 2 out]
        n293 = local write "USE_Func_ext"("" ("Func List 3")) -> ()
        n294 = property on="USE_Func_ext" class="CmbBox"("Strings And Values[]"=cluster{"String":string, "Value":string}[] [] ("문자열과 값[]")) -> ()  [unwired: 2 in, 2 out]
        n295 = Less Than 0?(x=w491) -> (x < 0?=w492:bool)
        n296 = call <vilib>:"Clear Errors.vi"("error in (no error)"=w472) -> ("error out"=w501:errorcluster)  [unwired: 5 in, 1 out]
        n297 = Select(t=T6."Disabled and Grayed Out" ("비활성화"), s=w492, f=T6."Enabled" ("비활성화")) -> (s? t:f=w495:T6)
        n298 = call <vilib>:"Unset Busy.vi"("error in (no error)"=w501) -> ("error out"=w502:errorcluster)  [unwired: 10 in]
        n299 = property on="PROC_절차생성" class="Bool"("DisabledEnum"=w495) -> ()  [unwired: 2 in, 2 out]
        n300 = Merge Errors(w502, w472) -> (w479:errorcluster)
        n301 = call "Enqueue Message.vi"("에러 입력(에러 없음)"=w479, "값"=w448, "메세지"="사이즈조정", "큐 입력"=w478) -> ("에러 출력"=w469:errorcluster, "큐 출력"=w467:refnum<queue>)  [unwired: 6 in]
        n302 = call "Enqueue Message.vi"("에러 입력(에러 없음)"=w469, "메세지"="탭변경", "큐 입력"=w467) -> ("에러 출력"=w468:errorcluster)  [unwired: 7 in, 1 out]
      }
      frame "에러" {
        n303 = Variant To Data(type=errorcluster {"status"=FALSE, "code"=0, "source"=""} ("에러 출력"), Variant=w504) -> (data=w507:errorcluster, error out=w505:errorcluster)  [unwired: 1 in]
        n304 = call <vilib>:"General Error Handler.vi"("error in (no error)"=w507) -> ()  [unwired: 10 in, 5 out]
      }
      frame "사이즈조정" {
        w523 = refnum<vi> refnum ("Slide 입력")
        # "패널 크기 조정"
        n305 = Variant To Data(error in=w512, type=refnum<vi>[] [] ("추가된 배열"), Variant=w510) -> (data=w508:refnum<vi>[], error out=w511:errorcluster)
        n306 = control-ref of="PROC_등록요청LIST"() -> (w524:refnum<vi>)
        n307 = control-ref of="탭 컨트롤"() -> (w518:refnum<vi>)
        n308 = control-ref of="STDNAM List"() -> (w522:refnum<vi>)
        n309 = control-ref of="슬라이드"() -> (w517:refnum<vi>)
        n310 = control-ref of="PROC_새로고침"() -> (w525:refnum<vi>)
        n311 = control-ref of="STD_등록List 검색"() -> (w514:refnum<vi>)
        n312 = control-ref of="PROC_새로고침"() -> (w519:refnum<vi>)
        n313 = control-ref of="Func Ind"() -> (w521:refnum<vi>)
        n314 = control-ref of="CMC Update"() -> (w515:refnum<vi>)
        n315 = control-ref of="STD_temp_LIST"() -> (w513:refnum<vi>)
        n316 = Build Array(w514, w519, w523, w521, w523, w522, w515, w523, w514) -> (w520:refnum<vi>[])
        n317 = call "DBM Pannel Size.vi"("TBCALSTD_temp"=w513, "새로고침 2"=w525, "tbl 참조 배열"=w508, "모델등록요청LIST 2"=w524, "에러 입력"=w511, "참조 배열"=w520, "TabCtl 참조 번호"=w518, "Slide 입력"=w517) -> ("에러 출력"=w516:errorcluster)  [unwired: 3 in]
      }
      frame "탭변경" {
        # "탭 컨트롤 값 변경"
        n318 = local read "탭 컨트롤"() -> (w526:T1)
        n319 = case shown="\"기준기 DB\", \"기준기 DB항목명칭\"" w526 {
          tunnel: [T6."Disabled and Grayed Out" ("비활성화") T6."Enabled" ("비활성화")] -> w529
          frame "기준기 DB", "기준기 DB항목명칭" {
          }
          frame Default {
          }
        }
        n320 = property on="TOP_항목명" class="Ring (엄격한)"(error in=w528, "DisabledEnum"=w529) -> (error out=w527:errorcluster)  [unwired: 1 in, 1 out]
      }
      frame "항목변경" {
        # "항목명 선택"
        n321 = Variant To Data(error in=w536, type="", Variant=w535) -> (data=w532:string, error out=w534:errorcluster)
        n322 = local read "교정기능목록"() -> (w537:string[][])
        n323 = local read "SubVI List"() -> (w541:string[])
        n324 = Search 1D Array(1D array=w541, element=w532) -> (index of element=w542:i32)  [unwired: 1 in]
        n325 = call-poly "Data Classification.vi"("DATA 입력"=w537, "검색 문자열"=w532) -> ("DATA 출력"=w546:string[][])  [unwired: 5 in, 4 out]
        n326 = Index Array(array=w537, index (col) #1=2 ("비활성화된 인덱스 (열)"), index (col) #2=0 ("비활성화된 인덱스 (열)")) -> (element #1=w556:string[], element #2=w553:string[])  [unwired: 2 in]
        n327 = Less Than 0?(x=w542) -> (x < 0?=w543:bool)
        n328 = Search 1D Array(1D array=w553, element=w532) -> (index of element=w552:i32)  [unwired: 1 in]
        n329 = Select(t=T6."Disabled and Grayed Out" ("비활성화"), s=w543, f=T6."Enabled" ("비활성화")) -> (s? t:f=w544:T6)
        n330 = Index Array(array=w556, index=w552) -> (element=→"Func Ind":string)
        n331 = property on="PROC_절차생성" class="Bool"(error in=w534, "DisabledEnum"=w544) -> (error out=w557:errorcluster)  [unwired: 1 in, 1 out]
        n332 = Insert Into Array(array=w546, index (row)=0 ("인덱스 (행)"), new element=string[] ["", ""] ("새 원소/부분배열")) -> (w554:string[][])  [unwired: 1 in]
        n333 = for {
          tunnel: w554 -> [w561] mode=indexing
          tunnel: [w560] -> w555 mode=indexing
          n334 = Index Array(array=w561) -> (element #4=w558:string, element #5=w559:string)  [unwired: 5 in, 3 out]
          n335 = Bundle(w559, w558) -> (w560:cluster{string, string})  [unwired: 1 in]
        }
        n336 = property on="USE_Func_ext" class="CmbBox"(error in=w557, "Strings And Values[]"=w555, "Value"="") -> (error out=w548:errorcluster)  [unwired: 1 in, 1 out]
      }
      frame "DB조회" {
        w562 = FALSE ("Cal Date ok?")
        # "조회 버튼, STD_교정일자 선택, STD_등록 List box 선택"
        n337 = local read "STD_교정일자"() -> (w584:string)
        n338 = local read "USE_Func_ext"() -> (w577:string)
        n339 = local read "세부분류목록"() -> (w582:string[][])
        n340 = call "DBM Var to Data.vi"("에러 입력"=w570, "값"=w571) -> ("에러 출력"=w569:errorcluster, "데이터"=w568:T4)  [unwired: 8 in]
        n341 = local read "TOP_항목명"() -> (w579:u16)
        n342 = local read "Func Ind"() -> (w575:string)
        n343 = local read "Func"() -> (w592:string)
        n344 = local read "옵션"() -> (w591:string)
        n345 = To Long Integer(number=w579) -> (32bit integer=w581:i32)
        n346 = call <vilib>:"Trim Whitespace.vi"("string"="PROC MDL") -> ("trimmed string"=w590:string)  [unwired: 1 in]
        n347 = call <vilib>:"Trim Whitespace.vi"("string"=w591) -> ("trimmed string"=w589:string)  [unwired: 1 in]
        n348 = call <vilib>:"Trim Whitespace.vi"("string"=w592) -> ("trimmed string"=w588:string)  [unwired: 1 in]
        n349 = call <vilib>:"Trim Whitespace.vi"("string"="ISID") -> ("trimmed string"=w587:string)  [unwired: 1 in]
        n350 = call <vilib>:"Trim Whitespace.vi"("string"="STDNAM List") -> ("trimmed string"=w585:string)  [unwired: 1 in]
        n351 = call <vilib>:"Trim Whitespace.vi"("string"=w584) -> ("trimmed string"=w583:string)  [unwired: 1 in]
        n352 = call <vilib>:"Trim Whitespace.vi"("string"=w577) -> ("trimmed string"=w576:string)  [unwired: 1 in]
        n353 = call <vilib>:"Trim Whitespace.vi"("string"=w575) -> ("trimmed string"=w574:string)  [unwired: 1 in]
        n354 = To Upper Case(1:w587) -> (0:w593:string)
        n355 = control-ref of="STD_교정일자"() -> (w596:refnum<vi>)
        n356 = call <vilib>:"Set Busy.vi"("error in (no error)"=w569) -> ("error out"=w601:errorcluster)  [unwired: 9 in, 1 out]
        n357 = control-ref of="STD Update"() -> (w595:refnum<vi>)
        n358 = control-ref of="CMC Update"() -> (w594:refnum<vi>)
        n359 = Index Array(array=w582, index (row)=w581, index (col)=0 ("비활성화된 인덱스 (열)")) -> (element=w578:string)
        n360 = Bundle By Name(cluster=T7 {"사번"="", "등록번호"="", "업체명"="", "세부분류코드"="", "형식"="", "기기번호"="", "FUNC"="", "FUNC_EXT"="", "옵션"="", "추가문자열"="", "일자"="", "배열 1"=[], "배열 2"=[], "항목명"="", "문자열"="", "이름"=""} ("Query info"), "세부분류코드"=w578, "형식"=w590, "옵션"=w589, "FUNC"=w588, "등록번호"=w593, "추가문자열"=w585, "일자"=w583, "FUNC_EXT"=w576, "항목명"=w574) -> (w567:T7)
        n361 = Build Array(w596, w595, w594) -> (w572:refnum<vi>[])
        n362 = call "DBM inquiry.vi"("컨트롤 참조"=w572, "Query info"=w567, "에러 입력"=w601, "데이터"=w568) -> ("에러 출력"=w597:errorcluster, "None?"=w573:bool, "Data"=w599:string[][], "테이블 참조 출력"=w600:refnum<vi>, "데이터 out"=w566:T4)  [unwired: 3 in]
        n363 = case shown="거짓" w573 {
          tunnel: w597 -> [w610 w620]
          tunnel: w600 -> [w609 _]
          tunnel: w599 -> [w607 _]
          tunnel: [w608 w620] -> w598
          tunnel: w566 -> [w606 _]
          frame False {
            n364 = Unbundle By Name(w606) -> ("문자열"=w605:string)
            n365 = call-poly "Cell Spacing.vi"("error in"=w610, "Data in"=w607, "테이블 참조 in"=w609) -> ("error out"=w608:errorcluster)  [unwired: 6 in, 2 out]
            n366 = case shown="기본" w605 {
              tunnel: w607 -> [_ w613]
              frame Default {
              }
              frame "기준기 DB" {
                n367 = for {
                  tunnel: w613 -> [w618] mode=indexing
                  tunnel: [w614] -> w612 mode=indexing
                  n368 = Index Array(array=w618, index=35 ("인덱스")) -> (element=w616:string)
                  n369 = Decimal String To Number(string=w616) -> (number=w615:i32)  [unwired: 2 in, 1 out]
                  n370 = Equal To 0?(x=w615) -> (x = 0?=w614:bool)
                }
                n371 = Or Array Elements(Boolean array=w612) -> (logical OR=w611:bool)
                n372 = local write "STD_notuse"(w611) -> ()
              }
            }
          }
          frame True {
            n373 = One Button Dialog(message="조회결과 없음." ("메시지")) -> ()  [unwired: 1 in, 1 out]
          }
        }
        n374 = local write "Cal Date ok?"(w562) -> ()
        n375 = local write "STDDB ok?"(w562) -> ()
        n376 = call <vilib>:"Clear Errors.vi"("error in (no error)"=w598) -> ("error out"=w603:errorcluster)  [unwired: 5 in, 1 out]
        n377 = call <vilib>:"Unset Busy.vi"("error in (no error)"=w603) -> ("error out"=w604:errorcluster)  [unwired: 10 in]
        n378 = Merge Errors(w604, w598) -> (w602:errorcluster)
      }
      frame "DB등록" {
        # "등록 버튼, 등록요청 버튼"
        n379 = local read "STD_교정일자"() -> (w661:string)
        n380 = local read "USE_Func_ext"() -> (w640:string)
        n381 = local read "세부분류목록"() -> (w648:string[][])
        n382 = local read "STDNAM List"() -> (w641:string)
        n383 = local read "TOP_항목명"() -> (w645:u16)
        n384 = global read "Global_Cal Info.vi" "교정자정보"() -> (w663:cluster{"사번":string, "이름":string, "자격":string})
        n385 = local read "PROC MDL"() -> (w643:string)
        n386 = call "DBM Var to Data.vi"("에러 입력"=w625, "값"=w623) -> ("에러 출력"=w624:errorcluster, "데이터"=w622:T4)  [unwired: 8 in]
        n387 = local read "Func Ind"() -> (w659:string)
        n388 = local read "Func"() -> (w657:string)
        n389 = local read "옵션"() -> (w656:string)
        n390 = local read "ISID"() -> (w642:string)
        n391 = To Long Integer(number=w645) -> (32bit integer=w647:i32)
        n392 = call <vilib>:"Trim Whitespace.vi"("string"=w643) -> ("trimmed string"=w655:string)  [unwired: 1 in]
        n393 = call <vilib>:"Trim Whitespace.vi"("string"=w656) -> ("trimmed string"=w654:string)  [unwired: 1 in]
        n394 = call <vilib>:"Trim Whitespace.vi"("string"=w657) -> ("trimmed string"=w653:string)  [unwired: 1 in]
        n395 = call <vilib>:"Trim Whitespace.vi"("string"=w642) -> ("trimmed string"=w652:string)  [unwired: 1 in]
        n396 = call <vilib>:"Trim Whitespace.vi"("string"=w641) -> ("trimmed string"=w650:string)  [unwired: 1 in]
        n397 = call <vilib>:"Trim Whitespace.vi"("string"=w661) -> ("trimmed string"=w649:string)  [unwired: 1 in]
        n398 = call <vilib>:"Trim Whitespace.vi"("string"=w640) -> ("trimmed string"=w658:string)  [unwired: 1 in]
        n399 = call <vilib>:"Trim Whitespace.vi"("string"=w659) -> ("trimmed string"=w660:string)  [unwired: 1 in]
        n400 = Unbundle By Name(w663) -> ("이름"=w664:string)
        n401 = To Upper Case(1:w652) -> (0:w662:string)
        n402 = Index Array(array=w648, index (row)=w647, index (col)=0 ("비활성화된 인덱스 (열)")) -> (element=w644:string)
        n403 = control-ref of="슬라이드"() -> (w627:refnum<vi>)
        n404 = call <vilib>:"Set Busy.vi"("error in (no error)"=w624) -> ("error out"=w633:errorcluster)  [unwired: 9 in, 1 out]
        n405 = control-ref of="STD Update"() -> (w632:refnum<vi>)
        n406 = control-ref of="CMC Update"() -> (w631:refnum<vi>)
        n407 = Bundle By Name(cluster=T7 {"사번"="", "등록번호"="", "업체명"="", "세부분류코드"="", "형식"="", "기기번호"="", "FUNC"="", "FUNC_EXT"="", "옵션"="", "추가문자열"="", "일자"="", "배열 1"=[], "배열 2"=[], "항목명"="", "문자열"="", "이름"=""} ("Query info"), "세부분류코드"=w644, "형식"=w655, "옵션"=w654, "FUNC"=w653, "등록번호"=w662, "추가문자열"=w650, "일자"=w649, "FUNC_EXT"=w658, "항목명"=w660, "이름"=w664) -> (w626:T7)
        n408 = call "DB Open.vi"("에러 입력"=w633) -> ("에러 출력"=w629:errorcluster, "참조 번호 출력"=w630:T13)  [unwired: 9 in]
        n409 = Build Array(w632, w631) -> (w628:refnum<vi>[])
        n410 = call "DBM Insert Data.vi"("Slide 참조 번호"=w627, "Query info"=w626, "배열"=w628, "데이터"=w622, "에러 입력"=w629, "참조 번호 입력"=w630) -> ("에러 출력"=w621:errorcluster, "참조 번호 출력"=w636:T13)  [unwired: 4 in]
        n411 = case shown="에러 .." w621 {
          selector: w621 -> [w667 w671]
          tunnel: [w670 w674] -> w637
          tunnel: w636 -> [w669 w676]
          frame No Error {
            n412 = One Button Dialog(message="등록완료." ("메시지")) -> ()  [unwired: 1 in, 1 out]
            n413 = call <vilib>:"DB Tools Close Connection.vi"("error in (no error)"=w667, "connection reference"=w669) -> ("error out"=w670:errorcluster)  [unwired: 5 in]
          }
          frame Error {
            n414 = call <vilib>:"DB Tools Close Connection.vi"("error in (no error)"=errorcluster {"status"=FALSE, "code"=0, "source"=""}, "connection reference"=w676) -> ("error out"=w673:errorcluster)  [unwired: 5 in]
            n415 = Merge Errors(w671, w673) -> (w674:errorcluster)
            n416 = One Button Dialog(message="등록실패!!" ("메시지")) -> ()  [unwired: 1 in, 1 out]
          }
        }
        n417 = call <vilib>:"Clear Errors.vi"("error in (no error)"=w637) -> ("error out"=w638:errorcluster)  [unwired: 5 in, 1 out]
        n418 = call <vilib>:"Unset Busy.vi"("error in (no error)"=w638) -> ("error out"=w639:errorcluster)  [unwired: 10 in]
        n419 = Merge Errors(w639, w637) -> (w635:errorcluster)
        n420 = call "Enqueue Message.vi"("에러 입력(에러 없음)"=w635, "메세지"="Initialize", "큐 입력"=w665) -> ("에러 출력"=w666:errorcluster)  [unwired: 7 in, 1 out]
      }
      frame "DB삭제" {
        # "삭제 버튼, 요청삭제 버튼"
        n421 = call "DBM Var to Data.vi"("에러 입력"=w716, "값"=w715) -> ("에러 출력"=w710:errorcluster, "데이터"=w702:T4)  [unwired: 8 in]
        n422 = local read "STD_교정일자"() -> (w689:string)
        n423 = local read "USE_Func_ext"() -> (w679:string)
        n424 = local read "세부분류목록"() -> (w687:string[][])
        n425 = local read "STDNAM List"() -> (w680:string)
        n426 = local read "TOP_항목명"() -> (w684:u16)
        n427 = local read "PROC MDL"() -> (w682:string)
        n428 = local read "Func Ind"() -> (w699:string)
        n429 = local read "Func"() -> (w697:string)
        n430 = local read "옵션"() -> (w696:string)
        n431 = local read "ISID"() -> (w681:string)
        n432 = call <vilib>:"Set Busy.vi"("error in (no error)"=w710) -> ("error out"=w705:errorcluster)  [unwired: 9 in, 1 out]
        n433 = To Long Integer(number=w684) -> (32bit integer=w686:i32)
        n434 = call <vilib>:"Trim Whitespace.vi"("string"=w682) -> ("trimmed string"=w695:string)  [unwired: 1 in]
        n435 = call <vilib>:"Trim Whitespace.vi"("string"=w696) -> ("trimmed string"=w694:string)  [unwired: 1 in]
        n436 = call <vilib>:"Trim Whitespace.vi"("string"=w697) -> ("trimmed string"=w693:string)  [unwired: 1 in]
        n437 = call <vilib>:"Trim Whitespace.vi"("string"=w681) -> ("trimmed string"=w692:string)  [unwired: 1 in]
        n438 = call <vilib>:"Trim Whitespace.vi"("string"=w680) -> ("trimmed string"=w690:string)  [unwired: 1 in]
        n439 = call <vilib>:"Trim Whitespace.vi"("string"=w689) -> ("trimmed string"=w688:string)  [unwired: 1 in]
        n440 = call <vilib>:"Trim Whitespace.vi"("string"=w679) -> ("trimmed string"=w698:string)  [unwired: 1 in]
        n441 = call <vilib>:"Trim Whitespace.vi"("string"=w699) -> ("trimmed string"=w700:string)  [unwired: 1 in]
        n442 = To Upper Case(1:w692) -> (0:w701:string)
        n443 = Index Array(array=w687, index (row)=w686, index (col)=0 ("비활성화된 인덱스 (열)")) -> (element=w683:string)
        n444 = Bundle By Name(cluster=T7 {"사번"="", "등록번호"="", "업체명"="", "세부분류코드"="", "형식"="", "기기번호"="", "FUNC"="", "FUNC_EXT"="", "옵션"="", "추가문자열"="", "일자"="", "배열 1"=[], "배열 2"=[], "항목명"="", "문자열"="", "이름"=""} ("Query info"), "세부분류코드"=w683, "형식"=w695, "옵션"=w694, "FUNC"=w693, "등록번호"=w701, "추가문자열"=w690, "일자"=w688, "FUNC_EXT"=w698, "항목명"=w700) -> (w678:T7)
        n445 = call "DB Open.vi"("에러 입력"=w705) -> ("에러 출력"=w704:errorcluster, "참조 번호 출력"=w703:T13)  [unwired: 9 in]
        n446 = call "DBM Delete Data.vi"("Query info"=w678, "데이터"=w702, "에러 입력"=w704, "참조 번호 입력"=w703) -> ("에러 출력"=w677:errorcluster, "참조 번호 출력"=w712:T13)  [unwired: 5 in, 1 out]
        n447 = case shown="에러 없음" w677 {
          selector: w677 -> [w717 w721]
          tunnel: [w720 w723] -> w711
          tunnel: w712 -> [w719 w726]
          frame No Error {
            n448 = One Button Dialog(message="삭제완료." ("메시지")) -> ()  [unwired: 1 in, 1 out]
            n449 = call <vilib>:"DB Tools Close Connection.vi"("error in (no error)"=w717, "connection reference"=w719) -> ("error out"=w720:errorcluster)  [unwired: 5 in]
          }
          frame Error {
            n450 = call <vilib>:"DB Tools Close Connection.vi"("error in (no error)"=errorcluster {"status"=FALSE, "code"=0, "source"=""}, "connection reference"=w726) -> ("error out"=w724:errorcluster)  [unwired: 5 in]
            n451 = One Button Dialog(message="삭제실패!!" ("메시지")) -> ()  [unwired: 1 in, 1 out]
            n452 = Merge Errors(w721, w724) -> (w723:errorcluster)
          }
        }
        n453 = call <vilib>:"Clear Errors.vi"("error in (no error)"=w711) -> ("error out"=w713:errorcluster)  [unwired: 5 in, 1 out]
        n454 = call <vilib>:"Unset Busy.vi"("error in (no error)"=w713) -> ("error out"=w714:errorcluster)  [unwired: 10 in]
        n455 = Merge Errors(w714, w711) -> (w708:errorcluster)
        n456 = call "Enqueue Message.vi"("에러 입력(에러 없음)"=w708, "메세지"="Initialize", "큐 입력"=w706) -> ("에러 출력"=w707:errorcluster)  [unwired: 7 in, 1 out]
      }
      frame "파일생성" {
        # "파일생성 버튼"
        n457 = Variant To Data(error in=w731, type=refnum<vi> refnum ("임의의 데이터"), Variant=w730) -> (data=w727:refnum<vi>, error out=w729:errorcluster)
        n458 = call <vilib>:"Set Busy.vi"("error in (no error)"=w729) -> ("error out"=w735:errorcluster)  [unwired: 9 in, 1 out]
        n459 = property class="Tbl (엄격한)"(reference=w727, error in=w735) -> (reference out=w732:refnum<vi>, "Value"=w734:string[][])  [unwired: 1 out]
        n460 = Empty Array?(array=w734) -> (empty?=w733:bool)
        n461 = case shown="거짓" w733 {
          tunnel: [w744 w759] -> w736
          tunnel: w735 -> [w742 w759]
          tunnel: w732 -> [w737 _]
          frame False {
            n462 = call "DBM File Save.vi"("에러 입력"=w742, "Table 입력"=w737) -> ("에러 출력"=w739:errorcluster, "File path"=w743:path)  [unwired: 8 in]
            n463 = call <vilib>:"Clear Errors.vi"("error in (no error)"=w739) -> ("error out"=w740:errorcluster)  [unwired: 5 in, 1 out]
            n464 = call <vilib>:"Unset Busy.vi"("error in (no error)"=w740) -> ("error out"=w741:errorcluster)  [unwired: 10 in]
            n465 = Merge Errors(w741, w739) -> (w738:errorcluster)
            n466 = case shown="에러" w738 {
              selector: w738 -> [w746 _]
              tunnel: [w746 w750] -> w744
              tunnel: w743 -> [_ w748]
              frame No Error {
                n467 = One Button Dialog(message="파일저장 완료." ("메시지")) -> ()  [unwired: 1 in, 1 out]
              }
              frame Error {
                n468 = Strip Path(path=w748) -> (name=w747:string)  [unwired: 1 out]
                n469 = Path To String(path=w748) -> (string=w749:string)
                n470 = xnode "에러 링"("파라미터 0"=w747, "파라미터 1"=w749) -> ("에러 출력"=w750:errorcluster)
              }
            }
          }
          frame True {
            n471 = One Button Dialog(message="데이터가 없습니다." ("메시지")) -> ()  [unwired: 1 in, 1 out]
          }
        }
      }
      frame "테이블초기화" {
        # "초기화 버튼"
        n472 = Variant To Data(error in=w765, type=refnum<vi>[] [] ("추가된 배열"), Variant=w764) -> (data=w763:refnum<vi>[], error out=w762:errorcluster)
        n473 = for {
          tunnel: w763 -> [w771] mode=indexing
          shift-right: [w767] -> w761
          shift-left: w762 -> [w768]
          n474 = property class="Tbl (엄격한)"(reference=w771, error in=w768, "Value"=string[][] [] ("값"), "Index Values"=T8 {"Row"=0, "Column"=0} ("인덱스 값")) -> (error out=w767:errorcluster)  [unwired: 1 out]
        }
      }
      frame "종료" {
        # "종료, 창닫기"
        n475 = Generate User Event(user event=w774, event data cluster=TRUE) -> (error out=w779:errorcluster)  [unwired: 2 in, 1 out]
        n476 = Release Queue(queue=w773, error in (no error)=w778) -> (error out=w772:errorcluster)  [unwired: 1 in, 2 out]
        n477 = Merge Errors(w779, w772) -> (w777:errorcluster)
      }
      frame "기준기성적서파일열기" {
        # "STD File Path 변경, STD RE 버튼"
        n478 = Variant To Data(error in=w785, type=path "", Variant=w783) -> (data=w781:path, error out=w784:errorcluster)
        n479 = call <vilib>:"Set Busy.vi"("error in (no error)"=w784) -> ("error out"=w795:errorcluster)  [unwired: 9 in, 1 out]
        n480 = call <vilib>:"Create Report.vi"("window state (normal)"=T10."minimized", "report type"=Report_Type."Excel", "template (empty)"=w781, "error in (no error)"=w795) -> ("report out"=w797:refnum<class "NI_report.lvclass">)  [unwired: 10 in, 1 out]
        n481 = call <vilib>:"Excel Workbook Properties.vi"("report in"=w797, "error in (no error)"=w795) -> ("report out"=w796:refnum<class "NI_report.lvclass">, "worksheets count"=w787:i32, "error out"=w794:errorcluster)  [unwired: 10 in, 1 out]
        n482 = case shown="기본" w787 {
          selector: w787 -> [_ w826]
          tunnel: w796 -> [w807 w825]
          tunnel: w794 -> [w806 w817]
          tunnel: [w807 w823] -> w790
          tunnel: [w806 w820] -> w789
          tunnel: [0 ("index of element") w809] -> w780
          frame 1 {
          }
          frame Default {
            n483 = call <vilib>:"Clear Errors.vi"("error in (no error)"=w817) -> ("error out"=w818:errorcluster)  [unwired: 5 in, 1 out]
            n484 = call <vilib>:"Excel Get Excel Location.vi"("cell's name"="B3") -> ("row"=w815:i32, "column"=w814:i32)
            n485 = call <vilib>:"Unset Busy.vi"("error in (no error)"=w818) -> ("error out"=w819:errorcluster)  [unwired: 10 in]
            n486 = Merge Errors(w819, w817) -> (w816:errorcluster)
            n487 = Bundle("row"=w815, "column"=w814) -> (w812:cluster{"row":i32, "column":i32})  [unwired: 1 in]
            n488 = for {
              N: w826 -> [_]
              shift-right: [w847] -> w823
              shift-left: w825 -> [w850]
              shift-right: [w846] -> w824
              shift-left: w816 -> [w849]
              tunnel: w812 -> [w845]
              tunnel: [w844] -> w822 mode=indexing if=w840
              tunnel: [w842] -> w808 mode=indexing if=w840
              i -> [w848]
              n489 = call <vilib>:"Excel Get Worksheet.vi"("report in"=w850, "worksheet index (0)"=w848, "error in (no error)"=w849) -> ("report out"=w847:refnum<class "NI_report.lvclass">, "error out"=w846:errorcluster)  [unwired: 11 in]
              n490 = call-poly <vilib>:"Excel Get Data.vi"("report in"=w847, "data type"="", "start (0, 0)"=w845, "error in (no error)"=w846) -> ("data"=w842:string)  [unwired: 9 in, 2 out]
              n491 = Empty String/Path?(string/path=w842) -> (empty?=w841:bool)
              n492 = Build Array(w842) -> (w844:string[])
              n493 = Not(x=w841) -> (.not. x?=w840:bool)
            }
            n494 = Array Size(array=w808) -> (size(s)=w811:i32)
            n495 = case shown="기본" w811 {
              tunnel: "기준기성적서파일열기" ("Func in") -> [_ w839]
              tunnel: [w830 w838] -> w810
              tunnel: string[] ["등록번호"] ("Col Header in") -> [_ w837]
              tunnel: w824 -> [w830 w836]
              tunnel: w822 -> [_ w835]
              tunnel: w808 -> [_ w834]
              tunnel: [0 ("index of element") w832] -> w809
              tunnel: "등록번호 선택" ("리스트명") -> [_ w831]
              frame 1 {
              }
              frame Default {
                n496 = call "User select_listbox.vi"("리스트명"=w831, "error in"=w836, "Col Header in"=w837, "Data in"=w835, "Func in"=w839) -> ("error out"=w838:errorcluster, "Text out"=w833:string)  [unwired: 3 in, 2 out]
                n497 = Search 1D Array(1D array=w834, element=w833) -> (index of element=w832:i32)  [unwired: 1 in]
              }
            }
            n498 = call <vilib>:"Set Busy.vi"("error in (no error)"=w810) -> ("error out"=w820:errorcluster)  [unwired: 9 in, 1 out]
          }
        }
        n499 = control-ref of="STD_교정일자"() -> (w798:refnum<vi>)
        n500 = control-ref of="TBCALSTD"() -> (w799:refnum<vi>)
        n501 = call "DBM STD File Open.vi"("TBCALSTD"=w799, "교정일자"=w798, "에러 입력"=w789, "close report? (T)"="파일닫기?", "index (0)"=w780, "report out"=w790) -> ("에러 출력"=w788:errorcluster, "등록번호"=w792:string, "Cal Date ok?"=→"Cal Date ok?":bool, "STDDB ok?"=w793:bool)  [unwired: 2 in]
        "STDDB ok?" <- w793
        n502 = local write "STD_notuse"(w793) -> ()
        n503 = local write "ISID"(w792) -> ()
        n504 = call <vilib>:"Clear Errors.vi"("error in (no error)"=w788) -> ("error out"=w803:errorcluster)  [unwired: 5 in, 1 out]
        n505 = call <vilib>:"Unset Busy.vi"("error in (no error)"=w803) -> ("error out"=w804:errorcluster)  [unwired: 10 in]
        n506 = Merge Errors(w804, w788) -> (w802:errorcluster)
      }
      frame "기준기등록리스트검색" {
        # "STD 등록List 검색 버튼"
        n507 = call <vilib>:"Set Busy.vi"("error in (no error)"=w865) -> ("error out"=w864:errorcluster)  [unwired: 9 in, 1 out]
        n508 = control-ref of="STD_List box"() -> (w871:refnum<vi>)
        n509 = call "DB Open.vi"("에러 입력"=w864) -> ("에러 출력"=w859:errorcluster, "참조 번호 출력"=w858:T13)  [unwired: 9 in]
        n510 = Bundle By Name(cluster=T7 {"사번"="", "등록번호"="", "업체명"="", "세부분류코드"="", "형식"="", "기기번호"="", "FUNC"="", "FUNC_EXT"="", "옵션"="", "추가문자열"="", "일자"="", "배열 1"=[], "배열 2"=[], "항목명"="", "문자열"="", "이름"=""} ("Query info"), "추가문자열"="STDDB STD List") -> (w851:T7)
        n511 = call "DB Read Queries.vi"("Query info"=w851, "Query Command"=Cmd_Read_Query."기준기등록리스트 얻기", "에러 입력(에러 없음)"=w859, "참조 번호 입력"=w858) -> ("에러 출력"=w856:errorcluster, "Data"=w855:string[][], "참조 번호 출력"=w857:T13)  [unwired: 3 in, 2 out]
        n512 = call <vilib>:"DB Tools Close Connection.vi"("error in (no error)"=w856, "connection reference"=w857) -> ("error out"=w870:errorcluster)  [unwired: 5 in]
        n513 = call-poly "Cell Spacing.vi"("error in"=w870, "Data in"=w855, "여러열리스트박스 참조 in"=w871) -> ("error out"=w869:errorcluster)  [unwired: 7 in, 1 out]
        n514 = property on="TBCALSTD" class="Tbl (엄격한)"(error in=w869) -> (error out=w868:errorcluster, "Height"=w866:u32)  [unwired: 1 in, 1 out]
        n515 = property on="STD_List box" class="MCListbox (엄격한)"(error in=w868, "Height"=w866, "Visible"=TRUE ("보이기")) -> (error out=w861:errorcluster)  [unwired: 1 in, 1 out]
        n516 = call <vilib>:"Clear Errors.vi"("error in (no error)"=w861) -> ("error out"=w862:errorcluster)  [unwired: 5 in, 1 out]
        n517 = call <vilib>:"Unset Busy.vi"("error in (no error)"=w862) -> ("error out"=w863:errorcluster)  [unwired: 10 in]
        n518 = Merge Errors(w863, w861) -> (w860:errorcluster)
      }
      frame "기준기DB요청열기" {
        # "STD 요청 리스트 버튼"
        n519 = call <vilib>:"Set Busy.vi"("error in (no error)"=w873) -> ("error out"=w887:errorcluster)  [unwired: 9 in, 1 out]
        n520 = Bundle By Name(cluster=T7 {"사번"="", "등록번호"="", "업체명"="", "세부분류코드"="", "형식"="", "기기번호"="", "FUNC"="", "FUNC_EXT"="", "옵션"="", "추가문자열"="", "일자"="", "배열 1"=[], "배열 2"=[], "항목명"="", "문자열"="", "이름"=""} ("Query info"), "추가문자열"="기준기요청리스트") -> (w891:T7)
        n521 = call "DB Open.vi"("에러 입력"=w887) -> ("에러 출력"=w878:errorcluster, "참조 번호 출력"=w879:T13)  [unwired: 9 in]
        n522 = control-ref of="STD_temp_LIST"() -> (w882:refnum<vi>)
        n523 = call "DB Read Queries.vi"("Query info"=w891, "Query Command"=Cmd_Read_Query."기준기요청 얻기", "에러 입력(에러 없음)"=w878, "참조 번호 입력"=w879) -> ("에러 출력"=w880:errorcluster, "Data"=w883:string[][], "참조 번호 출력"=w881:T13)  [unwired: 3 in, 2 out]
        n524 = call <vilib>:"DB Tools Close Connection.vi"("error in (no error)"=w880, "connection reference"=w881) -> ("error out"=w884:errorcluster)  [unwired: 5 in]
        n525 = call-poly "Cell Spacing.vi"("error in"=w884, "Data in"=w883, "여러열리스트박스 참조 in"=w882) -> ("error out"=w885:errorcluster, "여러열리스트박스 참조 out"=w886:refnum<vi>)  [unwired: 7 in]
        n526 = property on="프로퍼티 노드" class="MCListbox"(reference=w886, error in=w885, "Visible"=TRUE ("보이기")) -> (error out=w890:errorcluster)  [unwired: 1 out]
        n527 = call <vilib>:"Clear Errors.vi"("error in (no error)"=w890) -> ("error out"=w888:errorcluster)  [unwired: 5 in, 1 out]
        n528 = call <vilib>:"Unset Busy.vi"("error in (no error)"=w888) -> ("error out"=w889:errorcluster)  [unwired: 10 in]
        n529 = Merge Errors(w889, w890) -> (w872:errorcluster)
      }
      frame "기준기DB요청선택" {
        # "STD 요청 리스트 선택"
        n530 = Variant To Data(error in=w897, type=0 ("STD_temp_LIST"), Variant=w895) -> (data=w893:i32, error out=w896:errorcluster)
        n531 = call <vilib>:"Set Busy.vi"("error in (no error)"=w896) -> ("error out"=w901:errorcluster)  [unwired: 9 in, 1 out]
        n532 = property on="STD_temp_LIST" class="MCListbox (엄격한)"(error in=w901, "Visible"=FALSE ("보이기")) -> (error out=w899:errorcluster, "ItemNames"=w900:string[][])  [unwired: 1 in, 1 out]
        n533 = case shown="기본" w893 {
          selector: w893 -> [_ w908]
          tunnel: w899 -> [w905 w929]
          tunnel: w900 -> [_ w926]
          tunnel: [w905 w909] -> w904
          frame -1 {
          }
          frame Default {
            n534 = Index Array(array=w926, index (row) #1=w908, index (col) #1=0 ("비활성화된 인덱스 (열)")) -> (element #1=w907:string, element #2=w913:string)  [unwired: 2 in]
            n535 = call "DB Open.vi"("에러 입력"=w929) -> ("에러 출력"=w928:errorcluster, "참조 번호 출력"=w931:T13)  [unwired: 9 in]
            n536 = Bundle By Name(cluster=T7 {"사번"="", "등록번호"="", "업체명"="", "세부분류코드"="", "형식"="", "기기번호"="", "FUNC"="", "FUNC_EXT"="", "옵션"="", "추가문자열"="", "일자"="", "배열 1"=[], "배열 2"=[], "항목명"="", "문자열"="", "이름"=""} ("Query info"), "등록번호"=w907, "항목명"="TEMP" ("옵션")) -> (w915:T7)
            n537 = local write "ISID"(w907) -> ()
            n538 = call "DB Read Queries.vi"("Query info"=w915, "Query Command"=Cmd_Read_Query."DB (기준기값) 얻기", "에러 입력(에러 없음)"=w928, "참조 번호 입력"=w931) -> ("에러 출력"=w919:errorcluster, "Data"=w922:string[][], "참조 번호 출력"=w917:T13)  [unwired: 3 in, 2 out]
            n539 = Bundle By Name(cluster=w915, "추가문자열"=w913) -> (w914:T7)
            n540 = call "DB Read Queries.vi"("Query info"=w914, "Query Command"=Cmd_Read_Query."DB (STDNAME) 얻기", "에러 입력(에러 없음)"=w919, "참조 번호 입력"=w917) -> ("에러 출력"=w918:errorcluster, "Data (0번행)"=w912:string[], "참조 번호 출력"=w916:T13)  [unwired: 3 in, 2 out]
            n541 = control-ref of="TBCALSTD"() -> (w921:refnum<vi>)
            n542 = Build Array (concatenate)(string[] ["번호", "등록번호", "기기명(종류)"], w912, string[] ["요청자", "요청일자"]) -> (w910:string[])
            n543 = call <vilib>:"DB Tools Close Connection.vi"("error in (no error)"=w918, "connection reference"=w916) -> ("error out"=w923:errorcluster)  [unwired: 5 in]
            n544 = call-poly "Cell Spacing.vi"("Col Header in"=w910, "error in"=w923, "Data in"=w922, "테이블 참조 in"=w921) -> ("error out"=w909:errorcluster)  [unwired: 5 in, 2 out]
          }
        }
        n545 = call <vilib>:"Clear Errors.vi"("error in (no error)"=w904) -> ("error out"=w902:errorcluster)  [unwired: 5 in, 1 out]
        n546 = call <vilib>:"Unset Busy.vi"("error in (no error)"=w902) -> ("error out"=w903:errorcluster)  [unwired: 10 in]
        n547 = Merge Errors(w903, w904) -> (w898:errorcluster)
      }
      frame "기준기교정값내용검토" {
        w939 = 0 ("비활성화된 인덱스 (행)")
        w954 = 34 ("비활성화된 인덱스 (열)")
        # "STD 확인 버튼"
        n548 = local read "TBCALSTD"() -> (w951:string[][])
        n549 = call <vilib>:"Set Busy.vi"("error in (no error)"=w937) -> ("error out"=w936:errorcluster)  [unwired: 9 in, 1 out]
        n550 = Index Array(array=w951, index (row) #1=w939, index (col) #1=w954, index (col) #2=w954, index (row) #3=w939, index (col) #3=1 ("비활성화된 인덱스 (열)")) -> (element #1=w953:string, element #2=w952:string[], element #3=w938:string)  [unwired: 1 in]
        n551 = call "DB Open.vi"("에러 입력"=w936) -> ("에러 출력"=w948:errorcluster, "참조 번호 출력"=w947:T13)  [unwired: 9 in]
        n552 = Bundle By Name(cluster=T7 {"사번"="", "등록번호"="", "업체명"="", "세부분류코드"="", "형식"="", "기기번호"="", "FUNC"="", "FUNC_EXT"="", "옵션"="", "추가문자열"="", "일자"="", "배열 1"=[], "배열 2"=[], "항목명"="", "문자열"="", "이름"=""} ("Query info"), "등록번호"=w938) -> (w941:T7)
        n553 = call-poly "Array Deduplication.vi"("배열 in"=w952) -> ("배열 out"=w957:string[])  [unwired: 9 in, 1 out]
        n554 = call "DB Read Queries.vi"("Query info"=w941, "Query Command"=Cmd_Read_Query."교정일자(CAMAS) 얻기", "에러 입력(에러 없음)"=w948, "참조 번호 입력"=w947) -> ("에러 출력"=w945:errorcluster, "Data (0번행)"=w944:string[], "참조 번호 출력"=w946:T13)  [unwired: 3 in, 2 out]
        n555 = Array Size(array=w957) -> (size(s)=w956:i32)
        n556 = Index Array(array=w944) -> (element=w943:string)  [unwired: 1 in]
        n557 = call <vilib>:"DB Tools Close Connection.vi"("error in (no error)"=w945, "connection reference"=w946) -> ("error out"=w933:errorcluster)  [unwired: 5 in]
        n558 = Equal?(x=w956, y=1) -> (x = y?=w955:bool)
        n559 = Empty Array?(array=w951) -> (empty?=w961:bool)
        n560 = Not(x=w961) -> (.not. x?=w960:bool)
        n561 = Equal?(x=w953, y=w943) -> (x = y?=w962:bool)
        n562 = And(x=w962, y=w955) -> (x .and. y?=w958:bool)
        n563 = call <vilib>:"Clear Errors.vi"("error in (no error)"=w933) -> ("error out"=w934:errorcluster)  [unwired: 5 in, 1 out]
        n564 = And(x=w960, y=w958) -> (x .and. y?=w959:bool)
        n565 = call <vilib>:"Unset Busy.vi"("error in (no error)"=w934) -> ("error out"=w935:errorcluster)  [unwired: 10 in]
        n566 = local write "STDDB ok?"(w959) -> ()
        n567 = local write "Cal Date ok?"(w958) -> ()
        n568 = Merge Errors(w935, w933) -> (w932:errorcluster)
      }
      frame "DB업데이트" {
        # "STD not use 버튼"
        n569 = call "DBM Var to Data.vi"("에러 입력"=w973, "값"=w971) -> ("에러 출력"=w972:errorcluster, "데이터"=w964:T4)  [unwired: 8 in]
        n570 = Unbundle By Name(w964) -> ("문자열"=w963:string)
        n571 = call <vilib>:"Set Busy.vi"("error in (no error)"=w972) -> ("error out"=w974:errorcluster)  [unwired: 9 in, 1 out]
        n572 = local read "ISID"() -> (w965:string)
        n573 = Bundle By Name(cluster=T7 {"사번"="", "등록번호"="", "업체명"="", "세부분류코드"="", "형식"="", "기기번호"="", "FUNC"="", "FUNC_EXT"="", "옵션"="", "추가문자열"="", "일자"="", "배열 1"=[], "배열 2"=[], "항목명"="", "문자열"="", "이름"=""} ("Query info"), "등록번호"=w965, "추가문자열"=w963) -> (w966:T7)
        n574 = call "DB Open.vi"("에러 입력"=w974) -> ("에러 출력"=w975:errorcluster, "참조 번호 출력"=w976:T13)  [unwired: 9 in]
        n575 = call "DB Write Queries.vi"("Query info"=w966, "COMMAND"=Cmd_Write_Query."TBCALSTD_MCT NOTUSE update", "에러 입력(에러 없음)"=w975, "참조 번호 입력"=w976) -> ("에러 출력"=w968:errorcluster, "참조 번호 출력"=w969:T13)  [unwired: 6 in]
        n576 = case shown="에러" w968 {
          selector: w968 -> [w984 w989]
          tunnel: [w987 w990] -> w981
          tunnel: w969 -> [w986 w993]
          frame No Error {
            n577 = call <vilib>:"DB Tools Close Connection.vi"("error in (no error)"=w984, "connection reference"=w986) -> ("error out"=w987:errorcluster)  [unwired: 5 in]
            n578 = One Button Dialog(message="업데이트완료." ("메시지")) -> ()  [unwired: 1 in, 1 out]
          }
          frame Error {
            n579 = call <vilib>:"DB Tools Close Connection.vi"("error in (no error)"=errorcluster {"status"=FALSE, "code"=0, "source"=""}, "connection reference"=w993) -> ("error out"=w991:errorcluster)  [unwired: 5 in]
            n580 = Merge Errors(w989, w991) -> (w990:errorcluster)
            n581 = One Button Dialog(message="업데이트실패!!" ("메시지")) -> ()  [unwired: 1 in, 1 out]
          }
        }
        n582 = call <vilib>:"Clear Errors.vi"("error in (no error)"=w981) -> ("error out"=w982:errorcluster)  [unwired: 5 in, 1 out]
        n583 = call <vilib>:"Unset Busy.vi"("error in (no error)"=w982) -> ("error out"=w983:errorcluster)  [unwired: 10 in]
        n584 = Merge Errors(w983, w981) -> (w979:errorcluster)
        n585 = call "Enqueue Message.vi"("에러 입력(에러 없음)"=w979, "메세지"="Initialize", "큐 입력"=w977) -> ("에러 출력"=w978:errorcluster)  [unwired: 7 in, 1 out]
      }
      frame "모델선택" {
        # "PROC 모델 선택"
        n586 = call "DBM Var to Data.vi"("에러 입력"=w1005, "값"=w1004) -> ("에러 출력"=w1003:errorcluster, "데이터"=w994:T4)  [unwired: 8 in]
        n587 = local read "PROC_모델 선택"() -> (w1010:string)
        n588 = while {
          shift-right: [w1016] -> _
          shift-left: w1010 -> [w1021]
          tunnel: [w1013] -> w1002 mode=indexing
          shift-right: [w1012] -> w996
          shift-left: w1003 -> [w1012]
          stop <- w1018 stop-if-true
          w1014 = "▶" ("검색 문자열/문자 (-)")
          n589 = call <vilib>:"Trim Whitespace.vi"("string"=w1021) -> ("trimmed string"=w1020:string)  [unwired: 1 in]
          n590 = Search/Split String(string=w1020, search string/char (-)=w1014) -> (substring before match=w1017:string, match + rest of string=w1015:string, offset of match=w1019:i32)  [unwired: 1 in]
          n591 = Less Than 0?(x=w1019) -> (x < 0?=w1018:bool)
          n592 = Search and Replace String(input string=w1015, search string=w1014) -> (result string=w1016:string)  [unwired: 6 in, 3 out]
          n593 = call <vilib>:"Trim Whitespace.vi"("string"=w1017) -> ("trimmed string"=w1013:string)  [unwired: 1 in]
        }
        n594 = local read "세부분류목록"() -> (w1001:string[][])
        n595 = Index Array(array=w1002) -> (element #1=w995:string, element #2=w1007:string, element #3=w1006:string)  [unwired: 3 in]
        n596 = Index Array(array=w1001, index (col)=0 ("비활성화된 인덱스 (열)")) -> (element=w999:string[])  [unwired: 1 in]
        n597 = Search 1D Array(1D array=w999, element=w995) -> (index of element=w998:i32)  [unwired: 1 in]
        n598 = local write "PROC MDL"(w1007) -> ()
        n599 = local write "옵션"(w1006) -> ()
        n600 = To Unsigned Word Integer(number=w998) -> (unsigned 16bit integer=w1011:u16)
        n601 = local write "TOP_항목명"(w1011) -> ()
        n602 = call "Enqueue Message.vi"("에러 입력(에러 없음)"=w996, "값"=w994, "메세지"="DB조회", "큐 입력"=w1008) -> ("에러 출력"=w1009:errorcluster)  [unwired: 6 in, 1 out]
      }
      frame "절차생성" {
        # "PROC 절차생성 버튼"
        n603 = Variant To Data(error in=w1025, type="", Variant=w1026) -> (data=w1023:string, error out=w1022:errorcluster)
        n604 = call "DBM Create Proc.vi"("에러 입력"=w1022, "세부분류번호"=w1023) -> ("에러 출력"=w1032:errorcluster)  [unwired: 9 in]
        n605 = call "DBM Reg Req.vi"("에러 입력(에러 없음)"=w1032) -> ("에러 출력"=w1028:errorcluster, "모델 요청 갯수"=w1030:u8, "기준기 요청 갯수"=w1031:u8, "모델요청"=w1027:string[][])  [unwired: 6 in, 1 out]
        n606 = local write "기준기등록요청"(w1031) -> ()
        n607 = local write "모델등록요청"(w1030) -> ()
        n608 = control-ref of="PROC_등록요청LIST"() -> (w1029:refnum<vi>)
        n609 = call-poly "Cell Spacing.vi"("error in"=w1028, "Data in"=w1027, "여러열리스트박스 참조 in"=w1029) -> ()  [unwired: 7 in, 2 out]
      }
      frame "모델검색" {
        # "PROC 모델 검색 버튼"
        n610 = local read "세부분류목록"() -> (w1050:string[][])
        n611 = local read "TOP_항목명"() -> (w1048:u16)
        n612 = call <vilib>:"Set Busy.vi"("error in (no error)"=w1039) -> ("error out"=w1038:errorcluster)  [unwired: 9 in, 1 out]
        n613 = local read "PROC MDL"() -> (w1047:string)
        n614 = call "DB Open.vi"("에러 입력"=w1038) -> ("에러 출력"=w1033:errorcluster, "참조 번호 출력"=w1056:T13)  [unwired: 9 in]
        n615 = local read "옵션"() -> (w1051:string)
        n616 = To Long Integer(number=w1048) -> (32bit integer=w1049:i32)
        n617 = local read "SubVI List"() -> (w1042:string[])
        n618 = call <vilib>:"Trim Whitespace.vi"("string"=w1047) -> ("trimmed string"=w1041:string)  [unwired: 1 in]
        n619 = call <vilib>:"Trim Whitespace.vi"("string"=w1051) -> ("trimmed string"=w1040:string)  [unwired: 1 in]
        n620 = Index Array(array=w1050, index (row)=w1049, index (col)=0 ("비활성화된 인덱스 (열)")) -> (element=w1034:string)
        n621 = Bundle By Name(cluster=T7 {"사번"="", "등록번호"="", "업체명"="", "세부분류코드"="", "형식"="", "기기번호"="", "FUNC"="", "FUNC_EXT"="", "옵션"="", "추가문자열"="", "일자"="", "배열 1"=[], "배열 2"=[], "항목명"="", "문자열"="", "이름"=""} ("Query info"), "세부분류코드"=w1034, "형식"=w1041, "옵션"=w1040) -> (w1044:T7)
        n622 = Search 1D Array(1D array=w1042, element=w1034) -> (index of element=w1043:i32)  [unwired: 1 in]
        n623 = Less Than 0?(x=w1043) -> (x < 0?=w1037:bool)
        n624 = call "DB Read Queries.vi"("Query info"=w1044, "Query Command"=Cmd_Read_Query."모델(모델검색) 얻기", "에러 입력(에러 없음)"=w1033, "참조 번호 입력"=w1056) -> ("에러 출력"=w1059:errorcluster, "Data"=w1057:string[][], "참조 번호 출력"=w1055:T13, "None?"=w1058:bool)  [unwired: 3 in, 1 out]
        n625 = call <vilib>:"DB Tools Close Connection.vi"("error in (no error)"=w1059, "connection reference"=w1055) -> ("error out"=w1060:errorcluster)  [unwired: 5 in]
        n626 = case shown="거짓" w1058 {
          tunnel: w1057 -> [w1066 _]
          tunnel: [w1065 _] -> w1053
          frame False {
            n627 = for {
              tunnel: w1066 -> [w1072] mode=indexing
              tunnel: [w1068] -> w1065 mode=indexing
              n628 = Index Array(array=w1072) -> (element #1=w1071:string, element #2=w1070:string, element #3=w1067:string)  [unwired: 3 in]
              n629 = Format Into String(format string="%s ▶ %s ▶ %s" ("포맷 문자열"), w1071, w1070, w1067) -> (resulting string=w1068:string)  [unwired: 2 in, 1 out]
            }
          }
          frame True {
            n630 = One Button Dialog(message="데이터가 없습니다." ("메시지")) -> ()  [unwired: 1 in, 1 out]
          }
        }
        n631 = control-ref of="PROC_절차생성"() -> (w1036:refnum<vi>)
        n632 = Build Array(w1036) -> (w1035:refnum<vi>[])
        n633 = call "Set State Controls.vi"("활성화 (F)"=w1037, "컨트롤 참조 배열 in"=w1035) -> ()  [unwired: 8 in, 2 out]
        n634 = Index Array(array=w1053) -> (element=w1052:string)  [unwired: 1 in]
        n635 = property on="PROC_모델 선택" class="CmbBox"(error in=w1060, "Strings[]"=w1053, "Value"=w1052) -> (error out=w1061:errorcluster)  [unwired: 1 in, 1 out]
        n636 = call <vilib>:"Clear Errors.vi"("error in (no error)"=w1061) -> ("error out"=w1062:errorcluster)  [unwired: 5 in, 1 out]
        n637 = call <vilib>:"Unset Busy.vi"("error in (no error)"=w1062) -> ("error out"=w1063:errorcluster)  [unwired: 10 in]
        n638 = Merge Errors(w1063, w1061) -> (w1064:errorcluster)
      }
      frame "등록요청내용 조회" {
        # "PROC 등록요청list 선택"
        n639 = Variant To Data(error in=w1125, type=string[] [], Variant=w1124) -> (data=w1122:string[], error out=w1114:errorcluster)
        n640 = Index Array(array=w1122, index #1=1 ("인덱스")) -> (element #1=w1120:string, element #3=w1085:string, element #4=w1084:string)  [unwired: 3 in, 1 out]
        n641 = call <vilib>:"Set Busy.vi"("error in (no error)"=w1114) -> ("error out"=w1113:errorcluster)  [unwired: 9 in, 1 out]
        n642 = Bundle By Name(cluster=T7 {"사번"="", "등록번호"="", "업체명"="", "세부분류코드"="", "형식"="", "기기번호"="", "FUNC"="", "FUNC_EXT"="", "옵션"="", "추가문자열"="", "일자"="", "배열 1"=[], "배열 2"=[], "항목명"="", "문자열"="", "이름"=""} ("Query info"), "세부분류코드"=w1120, "형식"=w1085, "옵션"=w1084, "추가문자열"="TEMP") -> (w1083:T7)
        n643 = call "DB Open.vi"("에러 입력"=w1113) -> ("에러 출력"=w1097:errorcluster, "참조 번호 출력"=w1096:T13)  [unwired: 9 in]
        n644 = local read "세부분류목록"() -> (w1078:string[][])
        n645 = call "DB Read Queries.vi"("Query info"=w1083, "Query Command"=Cmd_Read_Query."교정기능 항목명칭 얻기", "에러 입력(에러 없음)"=w1097, "참조 번호 입력"=w1096) -> ("에러 출력"=w1093:errorcluster, "Data (0번행)"=w1115:string[], "참조 번호 출력"=w1092:T13)  [unwired: 3 in, 2 out]
        n646 = Unbundle By Name(w1083) -> ("세부분류코드"=w1077:string, "형식"=w1076:string, "옵션"=w1075:string)
        n647 = call "DB Read Queries.vi"("Query info"=w1083, "Query Command"=Cmd_Read_Query."교정절차 얻기", "에러 입력(에러 없음)"=w1093, "참조 번호 입력"=w1092) -> ("에러 출력"=w1090:errorcluster, "Data"=w1119:string[][], "참조 번호 출력"=w1091:T13)  [unwired: 3 in, 2 out]
        n648 = Build Array (concatenate)(string[] ["번호", "소분류번호", "세부분류번호", "기기명", "형식", "옵션"], w1115) -> (w1100:string[])
        n649 = control-ref of="TBCALPROC"() -> (w1109:refnum<vi>)
        n650 = Index Array(array=w1078, index (col)=0 ("비활성화된 인덱스 (열)")) -> (element=w1080:string[])  [unwired: 1 in]
        n651 = Insert Into Array(array=w1100, new element=string[] ["요청자", "요청일자"]) -> (w1099:string[])  [unwired: 1 in]
        n652 = Search 1D Array(1D array=w1080, element=w1077) -> (index of element=w1081:i32)  [unwired: 1 in]
        n653 = call-poly "Cell Spacing.vi"("Col Header in"=w1099, "error in"=w1090, "Data in"=w1119, "테이블 참조 in"=w1109) -> ("error out"=w1089:errorcluster)  [unwired: 5 in, 2 out]
        n654 = Bundle By Name(cluster=w1083, "옵션"="") -> (w1102:T7)
        n655 = To Unsigned Word Integer(number=w1081) -> (unsigned 16bit integer=w1082:u16)
        n656 = local write "PROC MDL"(w1076) -> ()
        n657 = local write "옵션"(w1075) -> ()
        n658 = call "DB Read Queries.vi"("Query info"=w1102, "Query Command"=Cmd_Read_Query."모델(모델검색) 얻기", "에러 입력(에러 없음)"=w1089, "참조 번호 입력"=w1091) -> ("에러 출력"=w1087:errorcluster, "Data"=w1106:string[][], "참조 번호 출력"=w1088:T13, "None?"=w1101:bool)  [unwired: 3 in, 1 out]
        n659 = local write "TOP_항목명"(w1082) -> ()
        n660 = case shown="거짓" w1101 {
          frame False {
            n661 = One Button Dialog(message="유사한 모델이 존재 합니다. 확인 후 등록하세요." ("메시지")) -> ()  [unwired: 1 in, 1 out]
          }
          frame True {
          }
        }
        n662 = for {
          tunnel: w1106 -> [w1132] mode=indexing
          tunnel: [w1129] -> w1104 mode=indexing
          tunnel: "%s ▶ %s ▶ %s" ("포맷 문자열") -> [w1127]
          n663 = Index Array(array=w1132) -> (element #1=w1131:string, element #2=w1130:string, element #3=w1128:string)  [unwired: 3 in]
          n664 = Format Into String(format string=w1127, w1131, w1130, w1128) -> (resulting string=w1129:string)  [unwired: 2 in, 1 out]
        }
        n665 = call <vilib>:"DB Tools Close Connection.vi"("error in (no error)"=w1087, "connection reference"=w1088) -> ("error out"=w1095:errorcluster)  [unwired: 5 in]
        n666 = Index Array(array=w1104) -> (element=w1103:string)  [unwired: 1 in]
        n667 = property on="PROC_모델 선택" class="CmbBox"(error in=w1095, "Strings[]"=w1104, "Value"=w1103) -> (error out=w1094:errorcluster)  [unwired: 1 in, 1 out]
        n668 = call <vilib>:"Clear Errors.vi"("error in (no error)"=w1094) -> ("error out"=w1111:errorcluster)  [unwired: 5 in, 1 out]
        n669 = call <vilib>:"Unset Busy.vi"("error in (no error)"=w1111) -> ("error out"=w1112:errorcluster)  [unwired: 10 in]
        n670 = Merge Errors(w1112, w1094) -> (w1110:errorcluster)
      }
      frame "등록요청리스트 갱신" {
        # "PROC 새로고침 버튼"
        n671 = Bundle By Name(cluster=T7 {"사번"="", "등록번호"="", "업체명"="", "세부분류코드"="", "형식"="", "기기번호"="", "FUNC"="", "FUNC_EXT"="", "옵션"="", "추가문자열"="", "일자"="", "배열 1"=[], "배열 2"=[], "항목명"="", "문자열"="", "이름"=""} ("Query info"), "추가문자열"="기준기요청리스트") -> (w1136:T7)
        n672 = call "DB Open.vi"("에러 입력"=w1148) -> ("에러 출력"=w1140:errorcluster, "참조 번호 출력"=w1139:T13)  [unwired: 9 in]
        n673 = call "DB Read Queries.vi"("Query info"=w1136, "Query Command"=Cmd_Read_Query."기준기요청 얻기", "에러 입력(에러 없음)"=w1140, "참조 번호 입력"=w1139) -> ("에러 출력"=w1143:errorcluster, "Data"=→"Data":string[][], "참조 번호 출력"=w1144:T13)  [unwired: 3 in, 2 out]
        n674 = control-ref of="PROC_등록요청LIST"() -> (w1147:refnum<vi>)
        n675 = call "DB Read Queries.vi"("Query Command"=Cmd_Read_Query."모델(등록요청) 얻기", "에러 입력(에러 없음)"=w1143, "참조 번호 입력"=w1144) -> ("에러 출력"=w1146:errorcluster, "Data"=w1133:string[][], "참조 번호 출력"=w1145:T13)  [unwired: 4 in, 2 out]
        n676 = call <vilib>:"DB Tools Close Connection.vi"("error in (no error)"=w1146, "connection reference"=w1145) -> ("error out"=w1134:errorcluster)  [unwired: 5 in]
        n677 = call-poly "Cell Spacing.vi"("error in"=w1134, "Data in"=w1133, "여러열리스트박스 참조 in"=w1147) -> ("error out"=w1149:errorcluster)  [unwired: 7 in, 1 out]
      }
      frame "세부교정기능목록" {
        # "USE STD 세부교정기능 선택"
        n678 = local read "교정기능목록"() -> (w1156:string[][])
        n679 = local read "TOP_항목명"() -> (w1161:u16)
        n680 = local read "세부분류목록"() -> (w1159:string[][])
        n681 = Variant To Data(error in=w1166, type="", Variant=w1165) -> (data=w1162:string, error out=w1163:errorcluster)
        n682 = To Long Integer(number=w1161) -> (32bit integer=w1160:i32)
        n683 = Index Array(array=w1159, index (row)=w1160, index (col)=0 ("비활성화된 인덱스 (열)")) -> (element=w1157:string)
        n684 = call-poly "Data Classification.vi"("DATA 입력"=w1156, "검색 문자열"=w1157) -> ("DATA 출력"=w1155:string[][])  [unwired: 5 in, 4 out]
        n685 = call-poly "Data Classification.vi"("인덱스"=3, "DATA 입력"=w1155, "검색 문자열"=w1162) -> ("DATA 출력"=w1153:string[][])  [unwired: 4 in, 4 out]
        n686 = call <vilib>:"Set Busy.vi"("error in (no error)"=w1163) -> ("error out"=w1171:errorcluster)  [unwired: 9 in, 1 out]
        n687 = Index Array(array=w1153, index (row)=0 ("인덱스 (행)"), index (col)=1 ("비활성화된 인덱스 (열)")) -> (element=→"Func":string)
        n688 = call "DB Open.vi"("에러 입력"=w1171) -> ("에러 출력"=w1176:errorcluster, "참조 번호 출력"=w1175:T13)  [unwired: 9 in]
        n689 = call "DB Read Queries.vi"("Query Command"=Cmd_Read_Query."DB (기준기이름목록) 얻기", "에러 입력(에러 없음)"=w1176, "참조 번호 입력"=w1175) -> ("에러 출력"=w1174:errorcluster, "Data"=w1178:string[][], "참조 번호 출력"=w1173:T13)  [unwired: 4 in, 2 out]
        n690 = call <vilib>:"DB Tools Close Connection.vi"("error in (no error)"=w1174, "connection reference"=w1173) -> ("error out"=w1179:errorcluster)  [unwired: 5 in]
        n691 = Index Array(array=w1178, index (col)=0 ("비활성화된 인덱스 (열)")) -> (element=w1180:string[])  [unwired: 1 in]
        n692 = property on="STD List" class="CmbBox"(error in=w1179, "Strings[]"=w1180) -> (error out=w1168:errorcluster)  [unwired: 1 in, 1 out]
        n693 = call <vilib>:"Clear Errors.vi"("error in (no error)"=w1168) -> ("error out"=w1169:errorcluster)  [unwired: 5 in, 1 out]
        n694 = call <vilib>:"Unset Busy.vi"("error in (no error)"=w1169) -> ("error out"=w1170:errorcluster)  [unwired: 10 in]
        n695 = Merge Errors(w1170, w1168) -> (w1167:errorcluster)
      }
      frame "사용기준기추가" {
        # "USE STD 추가 버튼"
        n696 = local read "USE_Func_ext"() -> (w1211:string)
        n697 = Variant To Data(error in=w1208, type="", Variant=w1207) -> (data=w1204:string, error out=w1205:errorcluster)
        n698 = local read "Func"() -> (w1212:string)
        n699 = call <vilib>:"Trim Whitespace.vi"("string"=w1212) -> ("trimmed string"=w1210:string)  [unwired: 1 in]
        n700 = call <vilib>:"Trim Whitespace.vi"("string"=w1211) -> ("trimmed string"=w1209:string)  [unwired: 1 in]
        n701 = call <vilib>:"Set Busy.vi"("error in (no error)"=w1205) -> ("error out"=w1191:errorcluster)  [unwired: 9 in, 1 out]
        n702 = Bundle By Name(cluster=T7 {"사번"="", "등록번호"="", "업체명"="", "세부분류코드"="", "형식"="", "기기번호"="", "FUNC"="", "FUNC_EXT"="", "옵션"="", "추가문자열"="", "일자"="", "배열 1"=[], "배열 2"=[], "항목명"="", "문자열"="", "이름"=""} ("Query info"), "FUNC"=w1210, "FUNC_EXT"=w1209, "세부분류코드"=w1204) -> (w1181:T7)
        n703 = call "DB Open.vi"("에러 입력"=w1191) -> ("에러 출력"=w1203:errorcluster, "참조 번호 출력"=w1202:T13)  [unwired: 9 in]
        n704 = call "DB Read Queries.vi"("Query info"=w1181, "Query Command"=Cmd_Read_Query."교정기능 명칭 얻기", "에러 입력(에러 없음)"=w1203, "참조 번호 입력"=w1202) -> ("에러 출력"=w1200:errorcluster, "Data (0번행)"=w1197:string[], "참조 번호 출력"=w1199:T13)  [unwired: 3 in, 2 out]
        n705 = call <vilib>:"DB Tools Close Connection.vi"("error in (no error)"=w1200, "connection reference"=w1199) -> ("error out"=w1188:errorcluster)  [unwired: 5 in]
        n706 = local read "세부분류목록"() -> (w1186:string[][])
        n707 = Index Array(array=w1197) -> (element #2=w1196:string, element #4=w1195:string)  [unwired: 4 in, 2 out]
        n708 = property on="TOP_항목명" class="Ring (엄격한)"(error in=w1188) -> (error out=w1187:errorcluster, "Value"=w1185:u16)  [unwired: 1 in, 1 out]
        n709 = Index Array(array=w1186, index (row)=w1185, index (col)=0 ("비활성화된 인덱스 (열)")) -> (element=w1183:string)
        n710 = local read "TBUSESTD"() -> (w1192:string[][])
        n711 = Build Array(w1183, w1210, w1196, w1209, w1195, "STD List") -> (w1193:string[])
        n712 = call <vilib>:"Clear Errors.vi"("error in (no error)"=w1187) -> ("error out"=w1189:errorcluster)  [unwired: 5 in, 1 out]
        n713 = call <vilib>:"Unset Busy.vi"("error in (no error)"=w1189) -> ("error out"=w1190:errorcluster)  [unwired: 10 in]
        n714 = Insert Into Array(array=w1192, new element=w1193) -> (w1198:string[][])  [unwired: 2 in]
        n715 = local write "TBUSESTD"(w1198) -> ()
        n716 = Merge Errors(w1190, w1187) -> (w1213:errorcluster)
      }
    }
  }
  n717 = Merge Errors(w33, w30) -> (w32:errorcluster)
  n718 = call "Destroy User Event - Stop.vi"("에러 입력(에러 없음)"=w32, "사용자 이벤트 입력"=w18) -> ("에러 출력"=→"error out":errorcluster)  [unwired: 9 in]
